vi "VI Interference Konfig.vi"() -> ()   [LabVIEW 2020, in "EPA 1065.lvlib" / "Interference verificaton 1065-366.lvlib"]
uses:
  Interference verificaton 1065-366.lvlib
  Visualisierungs Elemente/Zahlen-Ausgabefeld.ctl
  ResultTable.ctl
  TestKonfig.ctl
  Modus.ctl
  TestSetting.ctl
  Seiten/System Einstellungen V2/Analysatoren.ctl
  Visualisierungs Elemente/String - Ausgabefeld.ctl
  Aktion Test.ctl
  Aktion FGV Interference.ctl
  Sprachverwaltung/FGV Aktion Tabelle zerlegen.ctl
  Seiten/FT-IR/FGV FT-IR Gasliste Aktionen.ctl
  Aktion Index uebersetzten.ctl
  Allgemeine VIs/Aktion Test Status.ctl
  Allgemeine VIs/Aktion Wertaenderung Gasliste.ctl
  Messdaten/Aktionen FGV Messdaten.ctl
  Funktionstasten/Zustaende.ctl
  Funktionstasten/Funktionstasten-Aktion.ctl
  <vilib>/Utility/miscctls.llb/LVRowAndColumnTypeDef.ctl
  Seiten/FT-IR/FGV FT-IR Parameter.vi
  Messdaten/Messdaten.lvlib
  Seiten/Grafik/Grafik.lvlib
  Allgemein/allgemeine Sub-VIs.lvlib
  Seiten/FT-IR/FT-IR.lvlib
  Sprachverwaltung/Sprachverwaltung.lvlib
  Funktionstasten/Funktionstasten.lvlib
  Linearisierung V2/Protokoll/Protokoll.lvlib
  Seiten/FT-IR/Span/Spanfaktor.lvlib
  EPA 1065.lvlib
  Seiten/System Einstellungen V2/System Einstellungen V2.lvlib
panel:
  in  "Systemeinstellung":bool caption="Gasliste geändert"
  out "[%]":sgl=120.0 caption="Querempfindlichkeit:" min=0 format="%#.6g"
  in  "Gasliste vergleichen":bool
  in  "Registerkarte":T1(tab)
  in  "TestSetting":T2={"Bearbeiter:"="", "Pfad:"=path "D:/IAG_Data/Log", "Textname:"="", "Analysator"=""}
  in  "TestKonfig":T4={"CH4:"=0, "Ethane:"=0, "NMHC:"=0, "NMNEHC:"=0, "Komp 1 aktiv:"=FALSE, "Komp 2 aktiv:"=FALSE, "Komp 3 aktiv:"=FALSE, "Komp 4 aktiv:"=FALSE, "Modus"=0, "CG Aufschaltzeit:"=120.0, "Interferent 1: CO2"=0, "Interferent 2: H2O"=0, "Interferent 3: CH4"=0, "Interferent 4: C2H6 / C3H8"=0, "Gasflaschen Nr.:"="", "Gasflaschen Nr.: 3"="", "Gasflaschen Nr.: 4"="", "Inter 1 aktiv"=FALSE, "Inter 2 aktiv"=FALSE, "Inter 3 aktiv"=FALSE, "Inter 4 aktiv"=FALSE, "Accuracy"="", "Accuracy 3"="", "Accuracy 4"="", "Konzentration 1:"=120.0, "Konzentration 2:"=120.0, "Konzentration 3:"=120.0, "Konzentration 4:"=120.0, "Flow weighted mean 1:"=0.0, "Flow weighted mean 2:"=0.0, "Flow weighted mean 3:"=0.0, "Flow weighted mean 4:"=0.0} {"Flow weighted mean 4:" min=0.0; "NMNEHC:" items=["NMNEHCD (3000)"]; "Flow weighted mean 3:" min=0.0; "Flow weighted mean 2:" min=0.0; "Flow weighted mean 1:" min=0.0; "NMHC:" items=["NMHCD (10000)"]; "Ethane:" items=["Ethane (1000) LP 191C"]; "CH4:" items=["CH4 (250) LP 191C (1of2)", "CH4 (5000) LP 191C (2of2)", "CH4 autorange (5000)"]; "Konzentration 4:" min=0.0; "Interferent 4: C2H6 / C3H8" items=["Ethane (1000) LP 191C", "Propane (200) LP 191C"]; "Konzentration 3:" min=0.0; "Interferent 3: CH4" items=["CH4 (250) LP 191C (1of2)", "CH4 (5000) LP 191C (2of2)", "CH4 autorange (5000)"]; "Konzentration 2:" min=0.0; "Interferent 2: H2O" items=["H2O% (30) LP 191C", "H2Oppm (300000)"]; "Konzentration 1:" min=0.0; "Interferent 1: CO2" items=["CO2 low% (4) LP 191C (2of2)", "CO2% (20) LP 191C (1of2)", "CO2% autorange (20)"]; "Modus" items=["Messen", "CG zu Entnahmestelle"]; "CG Aufschaltzeit:" min=60.0}
  in  "Speichern":bool
  out "Komponente 4S:":T6 caption="NMNEHC:"
  out "Komponente 4:":T7 caption="ppm" format="%#.2f"
  out "Komponente 3S:":T6 caption="NMHC:"
  out "Komponente 3:":T7 caption="ppm" format="%#.2f"
  out "Komponente 2S:":T6 caption="Ethane:"
  out "Komponente 2:":T7 caption="ppm" format="%#.2f"
  in  "Graph löschen":bool caption="Test Start"
  out "Interferent 4:":T6 caption="Interferent 3:"
  out "Interferent 4:":T7 caption="ppm" format="%#.2f"
  out "Interferent 3:":T6
  out "Interferent 3: 2":T7 caption="ppm" format="%#.2f"
  out "Interferent 2:":T6
  out "Interferent 2: 2":T7 caption="%" format="%#.2f"
  out "Interferent 1:":T6
  out "Interferent 1: 2":T7 caption="%" format="%#.2f"
  in  "Abbrechen":bool caption="Test Start"
  out "Testdauer":T7
  out "Stabilisierungszeit":T7
  out "Graph":waveform(dbl)[](graph)
  out "Status":string
  in  "Test Start":bool
  out "Komponente 1S:":T6 caption="CH4:"
  out "Komponente 1:":T7 caption="ppm" format="%#.2f"
  in  "Save to file":bool caption="PDF erstellen"
  out "Grenze in ppm:":sgl=2.0 min=0 format="%#.6g"
  out "[%]":sgl=2.0 caption="Grenze:" min=0 format="%#.6g"
  out "Konzentration Komponente":sgl=120.0 caption="Konzentration:" min=0
  out "Komponente:":T6 caption="ppm"
  out "max. Flow Weighted Mean:":T6 caption="ppm"
  out "Konzentration FlowWeightedMean":sgl=120.0 caption="Konzentration:" min=0 format="%#.2f"
  out "LIN Ausgabetabelle":T8
  in  "Daten löschen":bool caption="Test Start"
  in  "Print to PDF":bool caption="PDF erstellen"
  out "Tabelle 3":string[][](table)
  # "HC Querempfindlichkeitsnachweis 1065.366"
  # "Interference Test"
  # "Interference Verification"
  # "Einstellungen"
  # "Allgemeine Einstellungen"
  # "Protocol Settings"
  # "Test Einstellungen"
  # "Durchflussgewichteter Mittelwert:"
  # "Interferenten"
  # "sec."
  # "Test"
  # "Ergebnis"
  # "Analyse"
  # "Interferenz für Komponente:"
  # "Durchflussgewichteter Mittelwert:"
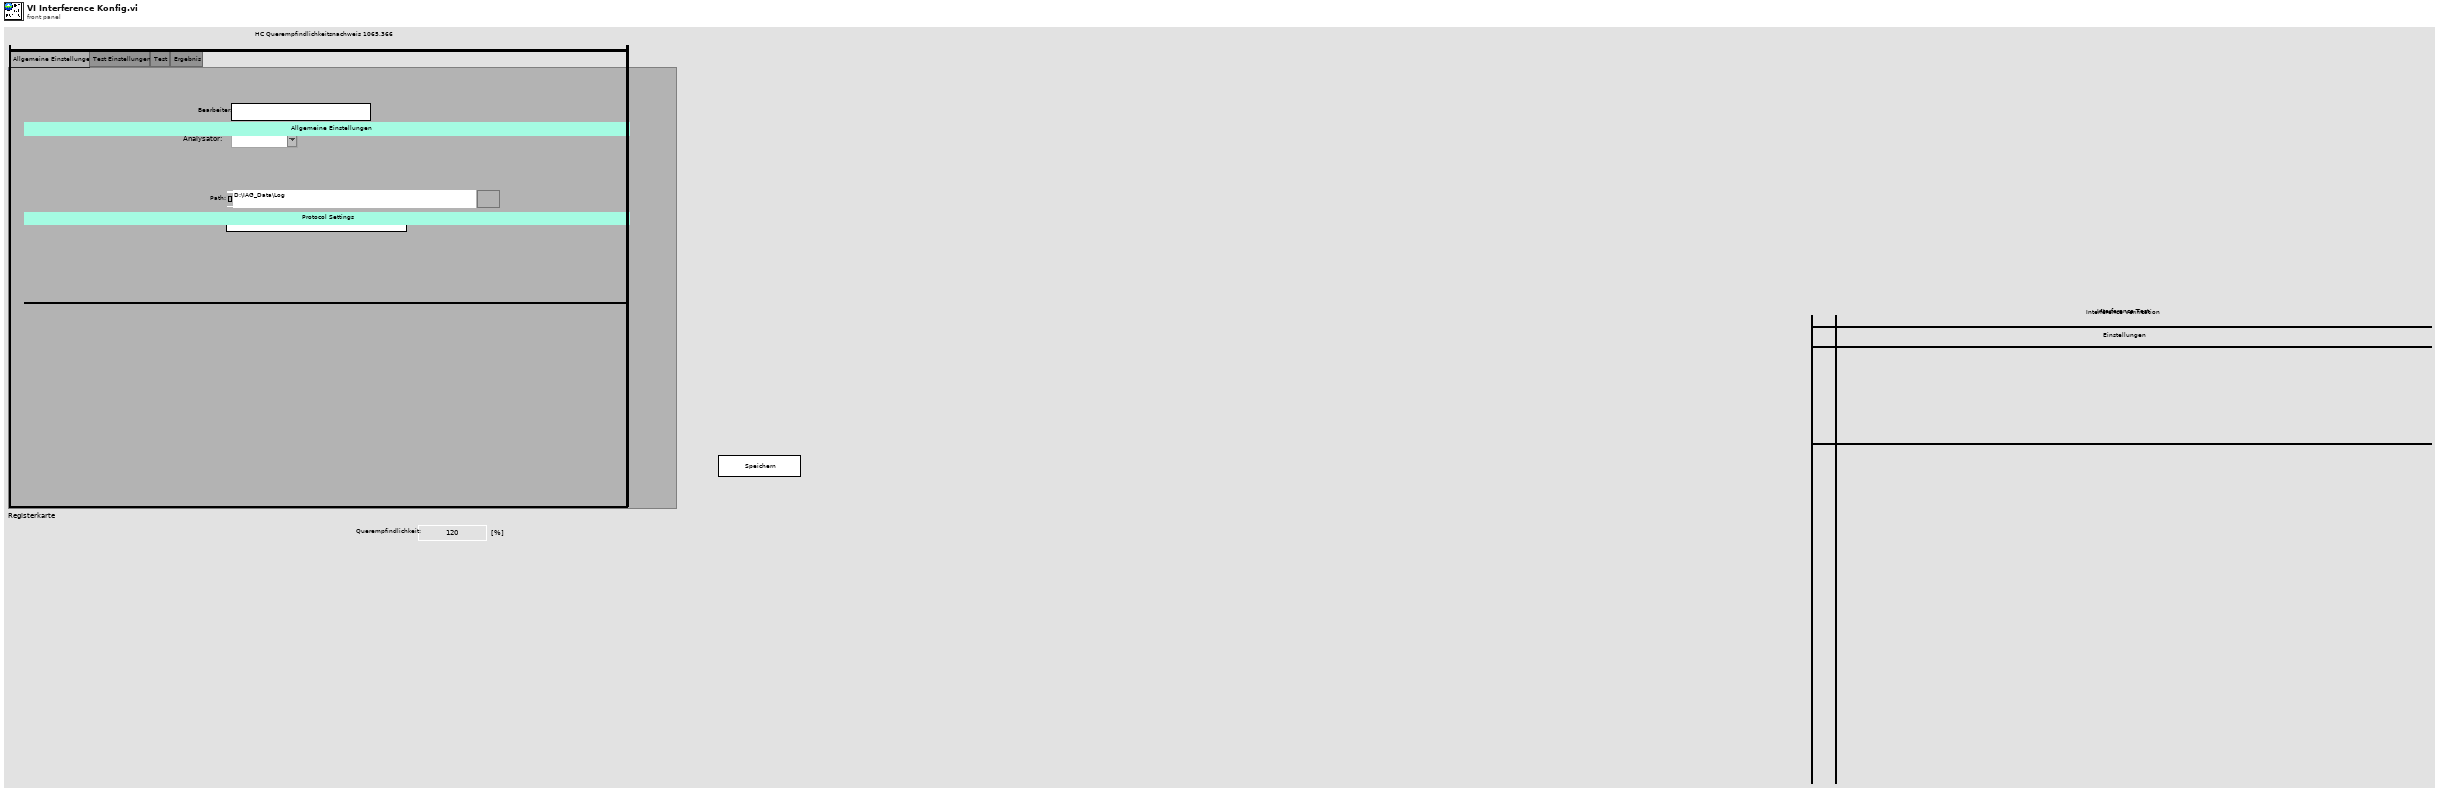
[diagram p1: front panel]
types:
  T1 = enum32{"General Settings", "Test Settings", "Test", "Result"}
  T2 = typedef "EPA 1065.lvlib/Interference verificaton 1065-366.lvlib/TestSetting.ctl" = cluster{"Bearbeiter:":string, "Pfad:":path, "Textname:":string, "Analysator":T3}
  T3 = typedef "System Einstellungen V2.lvlib/Analysatoren.ctl" = string
  T4 = typedef "EPA 1065.lvlib/Interference verificaton 1065-366.lvlib/TestKonfig.ctl" = cluster{"CH4:":u16, "Ethane:":u16, "NMHC:":u16, "NMNEHC:":u16, "Komp 1 aktiv:":bool, "Komp 2 aktiv:":bool, "Komp 3 aktiv:":bool, "Komp 4 aktiv:":bool, "Modus":T5, "CG Aufschaltzeit:":dbl, "Interferent 1: CO2":u16, "Interferent 2: H2O":u16, "Interferent 3: CH4":u16, "Interferent 4: C2H6 / C3H8":u16, "Gasflaschen Nr.:":string, "Gasflaschen Nr.: 3":string, "Gasflaschen Nr.: 4":string, "Inter 1 aktiv":bool, "Inter 2 aktiv":bool, "Inter 3 aktiv":bool, "Inter 4 aktiv":bool, "Accuracy":string, "Accuracy 3":string, "Accuracy 4":string, "Konzentration 1:":dbl, "Konzentration 2:":dbl, "Konzentration 3:":dbl, "Konzentration 4:":dbl, "Flow weighted mean 1:":dbl, "Flow weighted mean 2:":dbl, "Flow weighted mean 3:":dbl, "Flow weighted mean 4:":dbl}
  T5 = typedef "EPA 1065.lvlib/Interference verificaton 1065-366.lvlib/Modus.ctl" = u16
  T6 = typedef "String - Ausgabefeld.ctl" = string
  T7 = typedef "Zahlen-Ausgabefeld.ctl" = sgl
  T8 = typedef "EPA 1065.lvlib/Interference verificaton 1065-366.lvlib/ResultTable.ctl" = string[][]
  T9 = typedef "EPA 1065.lvlib/Interference verificaton 1065-366.lvlib/Aktion Test.ctl" = enum16{"Lesen", "ini", "ini - Konz", "Konzentration erreicht", "ini-warten", "ini-Warten-Stabil", "Warten-Stabil", "ini-warten-aufzeichnen", "Warten-Aufzeichnen", "aufzeichnen", "ini-wet", "ini - konz - wet", "Konzentration erreicht - wet", "ini - warten - wet", "warten - wet", "warten - aufzeichnen - wet", "Auswerten", "aufzeichnen - wet"}
  T10 = typedef "Sprachverwaltung.lvlib/FGV Aktion Tabelle zerlegen.ctl" = enum16{"laden", "vereinzeln", "speichern"}
  T11 = typedef "EPA 1065.lvlib/Interference verificaton 1065-366.lvlib/Aktion FGV Interference.ctl" = enum16{"Lesen", "TestKonfig", "TestSetting", "Einheiten", "Ergebnis", "Laden", "Tabelle", "Speichern", "löschen"}
  T12 = enum16{"Deutsch", "Englisch", "Französisch", "Italienisch"}
  T13 = enum8{"Enabled", "Disabled", "Disabled and Grayed Out"}
  T14 = typedef "EPA 1065.lvlib/Interference verificaton 1065-366.lvlib/Aktion Index uebersetzten.ctl" = enum16{"lesen", "schreiben", "auswerten"}
  T15 = typedef "FT-IR.lvlib/FGV FT-IR Gasliste Aktionen.ctl" = enum16{"lesen", "Gasliste FT-IR", "Gasliste ausgelesen", "laden", "speichern", "löschen"}
  T16 = typedef "EPA 1065.lvlib/Interference verificaton 1065-366.lvlib/Komponenten.ctl" = cluster{"Komponente":T6, "Komponente Index":i32, "Komponente 2":T6, "Komponente Index 2":i32, "Komponente 3":T6, "Komponente Index 3":i32, "Komponente 4":T6, "Komponente Index 4":i32, "Interferent 1":T6, "Interferent Index":i32, "Interferent 2":T6, "Interferent 2 Index":i32, "Interferent 3":T6, "Interferent 3 Index":i32, "Interferent 4":T6, "Interferent 4 Index":i32}
  T17 = typedef "EPA 1065.lvlib/Aktion Wertaenderung Gasliste.ctl" = enum16{"Init", "lesen", "Gasliste geändert", "ARN inaktiv", "LEAK inaktiv", "Interference 366 inaktiv", "T90 inaktiv", "Interference 375 inaktiv", "Chiller inaktiv", "FID O2 inaktiv", "FID Opti inaktiv", "Drift inaktiv", "Pre Test inaktiv", "LinV2 inaktiv", "HovaCAL Interference inaktiv"}
  T18 = typedef "EPA 1065.lvlib/Aktion Test Status.ctl" = enum16{"init", "lesen", "prüfen", "Interference 366", "Interference 375", "Chiller läuft", "Drift läuft", "Pre Test läuft", "FID Optimization läuft", "FID Interference läuft", "HovaCAL Interference", "LinV2"}
  T19 = typedef "Messdaten.lvlib/Aktionen FGV Messdaten.ctl" = enum16{"lesen", "schreiben", "löschen", "Mittelwerte", "Komponente"}
  T20 = typedef "Funktionstasten.lvlib/Funktionstasten-Aktion.ctl" = enum16{"Initialisieren", "Zustand setzen", "Taste gedrückt", "Fehler speichern", "Lesen", "Manuell", "Remote", "Bitparallel", "Samplepoint", "Zeit Prüfen", "reset Umschalten"}
  T21 = typedef "Funktionstasten.lvlib/Zustaende.ctl" = enum16{"Standby", "Pause", "Eco", "Messen", "Kalibrieren", "Spülen Filter", "Spülen Leitung", "Umgebungsluft", "0-Gas", "Cal-Gas", "CG zu PNS", "-------------", "Init 1", "Init 2", "Init 3", "Init 4", "Messen vorbereiten", "Messen durchführen", "Exit"}
  T22 = enum16{"open", "replace", "create", "open or create", "replace or create", "replace or create with confirmation"}
  T23 = typedef "LVRowAndColumnTypeDef.ctl" = cluster{"Row":i32, "Column":i32}
  T24 = typedef "EPA 1065.lvlib/Aktive Tests Cluster.ctl" = cluster{"ANR läuft":bool, "T90 läuft":bool, "Leak läuft":bool, "Interference 366 läuft":bool, "Interference 375 läuft":bool, "Chiller läuft":bool, "FID Interference läuft":bool, "FID optimization läuft":bool, "Drift läuft":bool, "Pre-test läuft":bool, "HovaCAL Interference läuft":bool, "LinV2 läuft":bool}
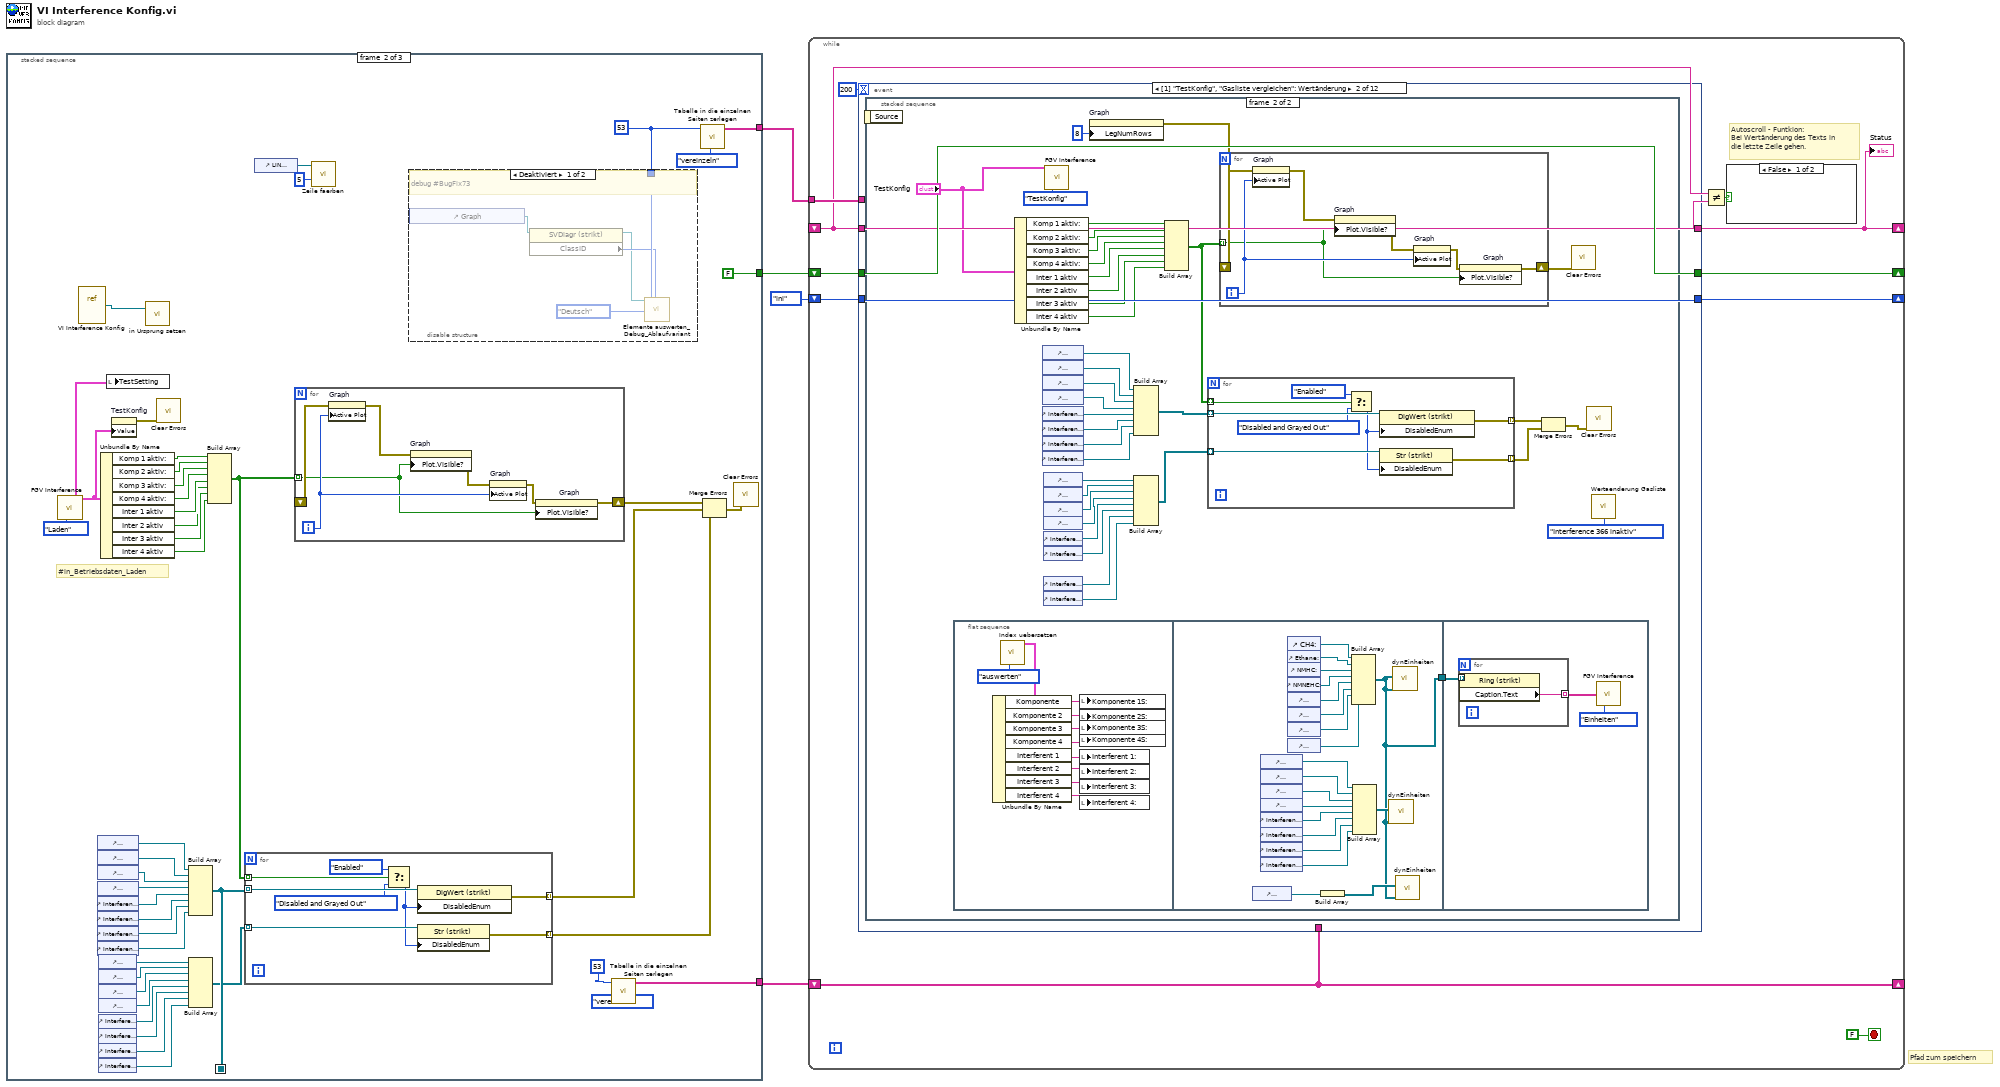
[diagram p0: block diagram]
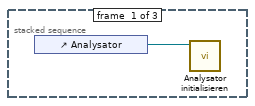
[diagram p2: hidden frame]
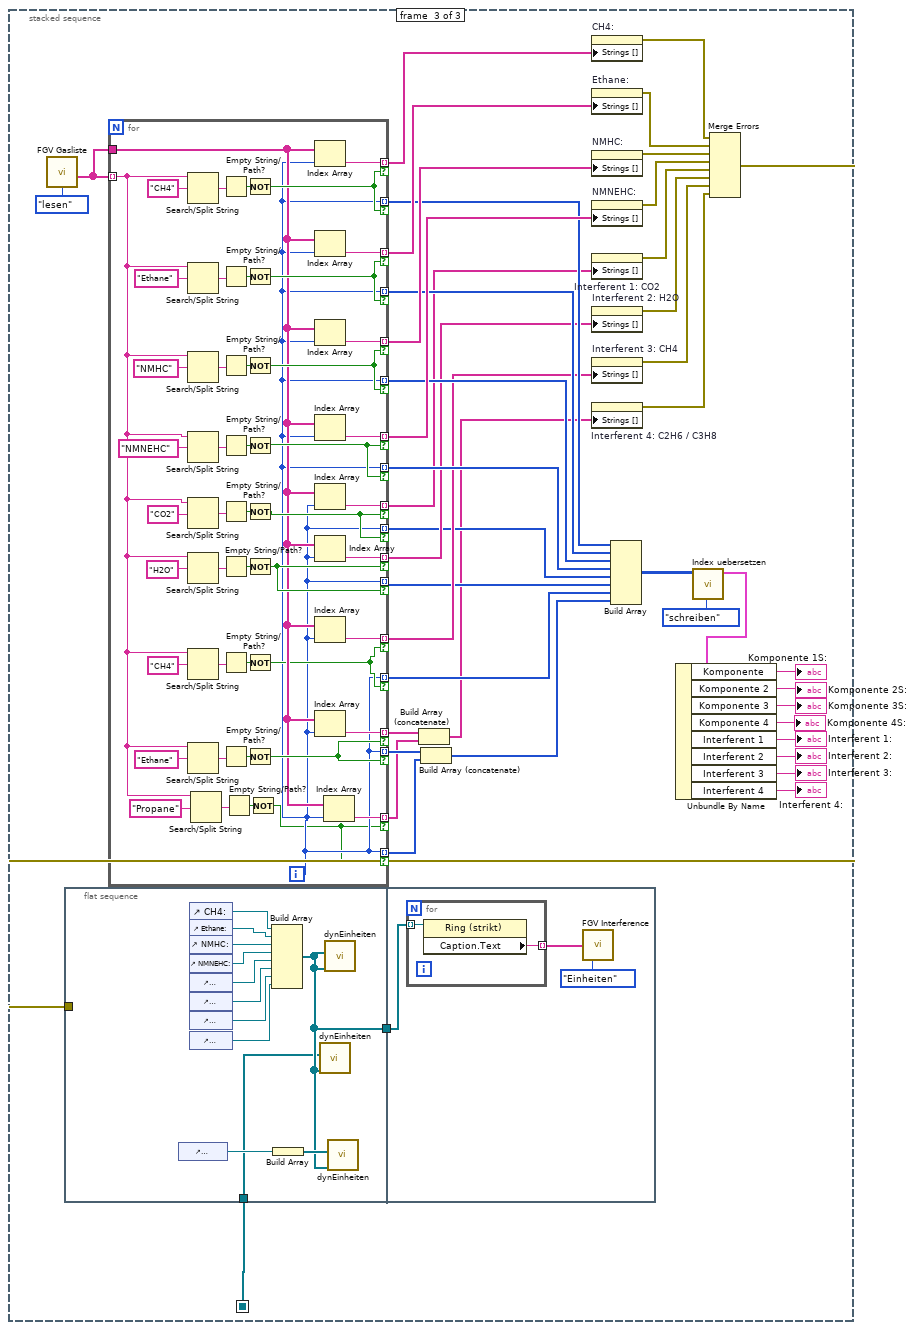
[diagram p4: hidden frame]
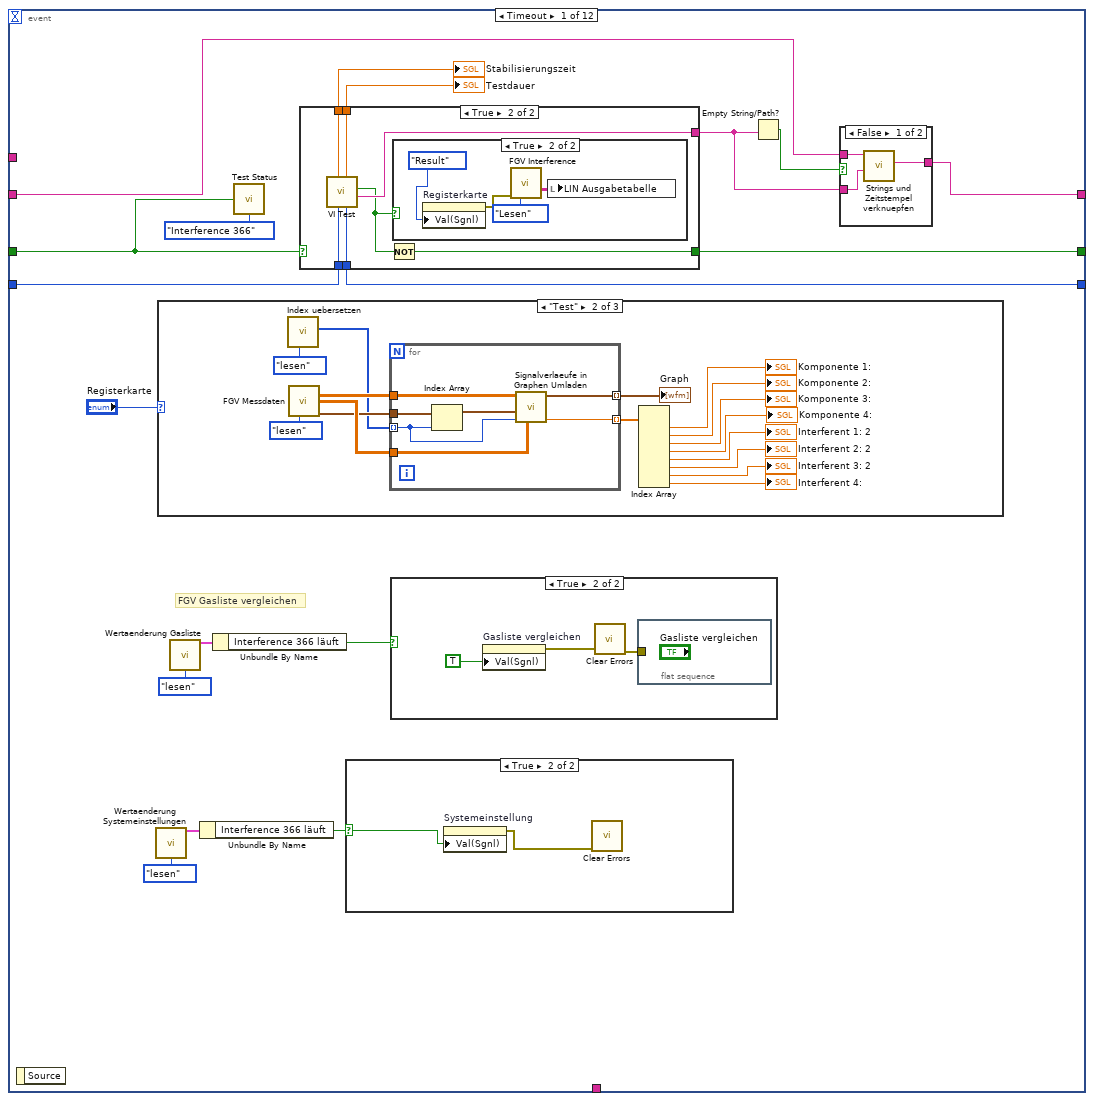
[diagram p5: hidden frame]
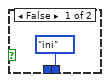
[diagram p10: hidden frame]
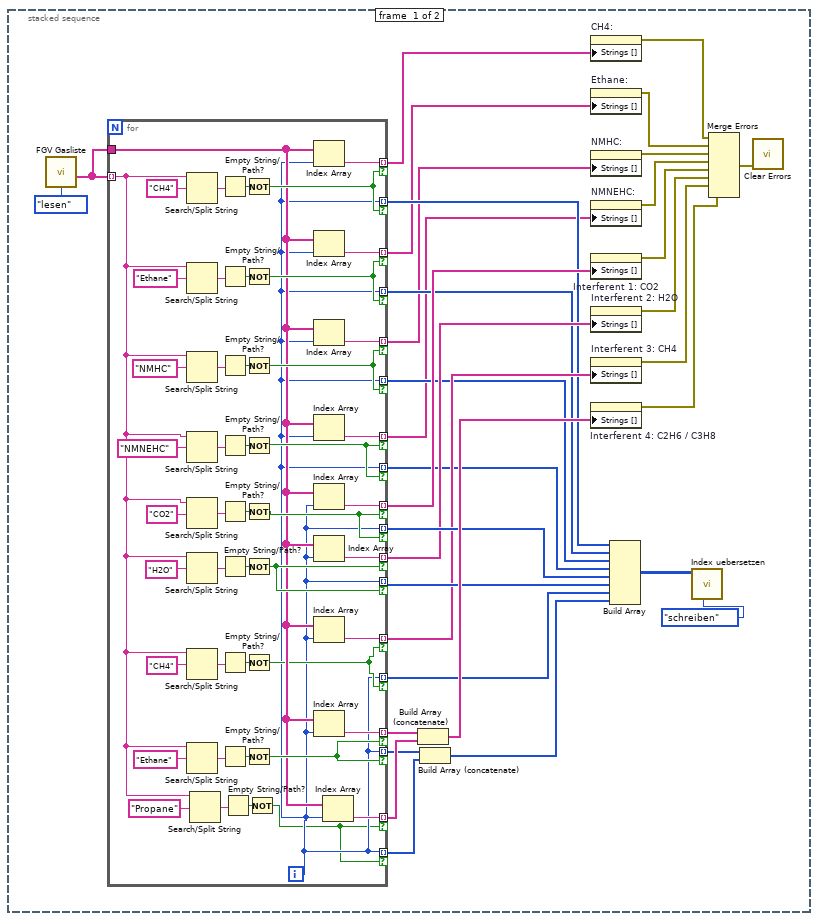
[diagram p13: hidden frame]
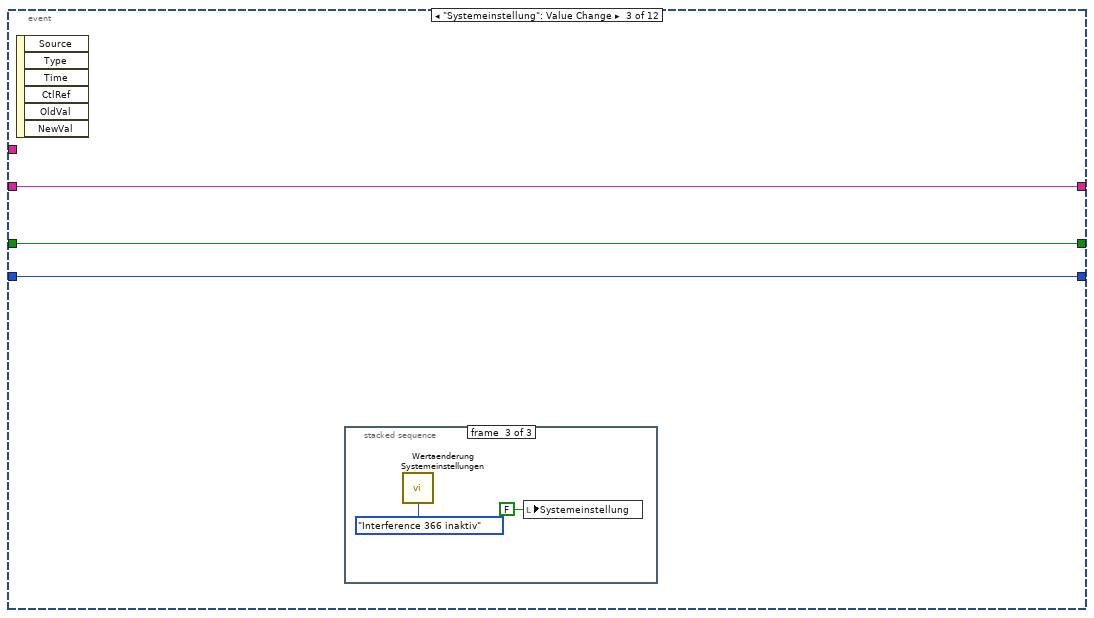
[diagram p14: hidden frame]
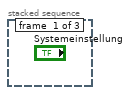
[diagram p15: hidden frame]
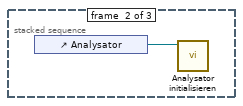
[diagram p16: hidden frame]
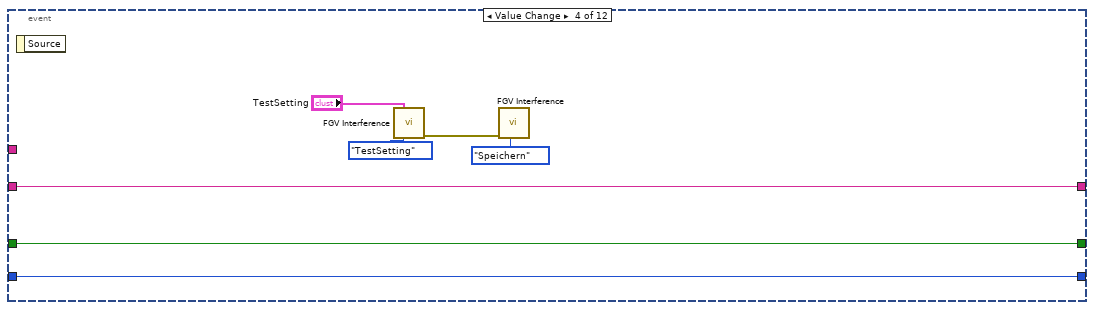
[diagram p17: hidden frame]
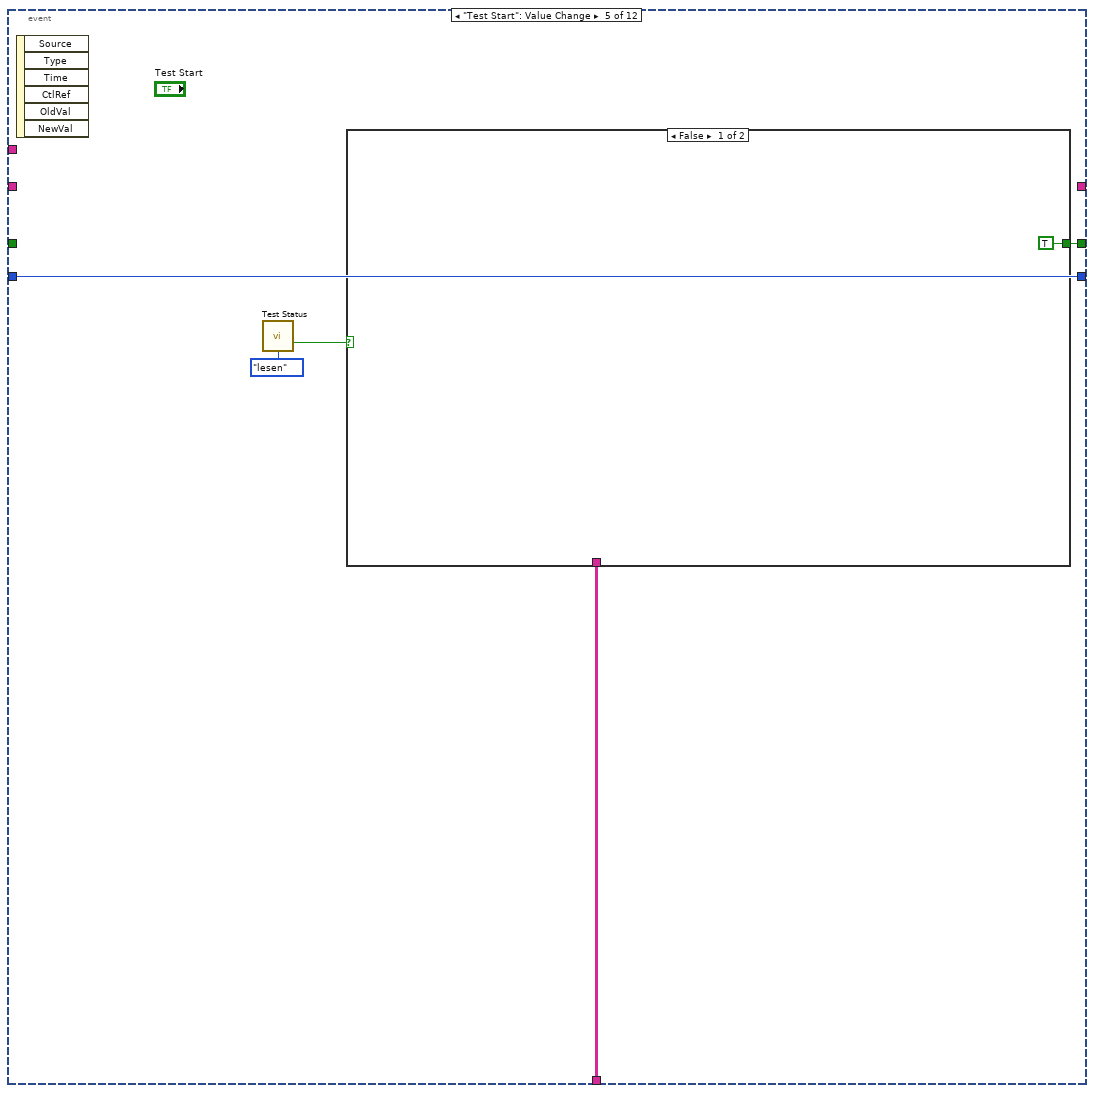
[diagram p18: hidden frame]
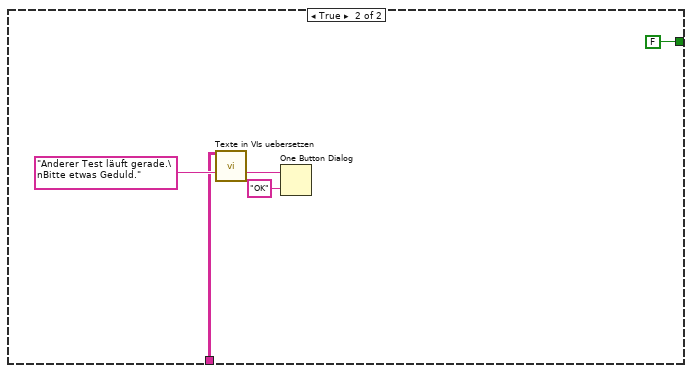
[diagram p19: hidden frame]
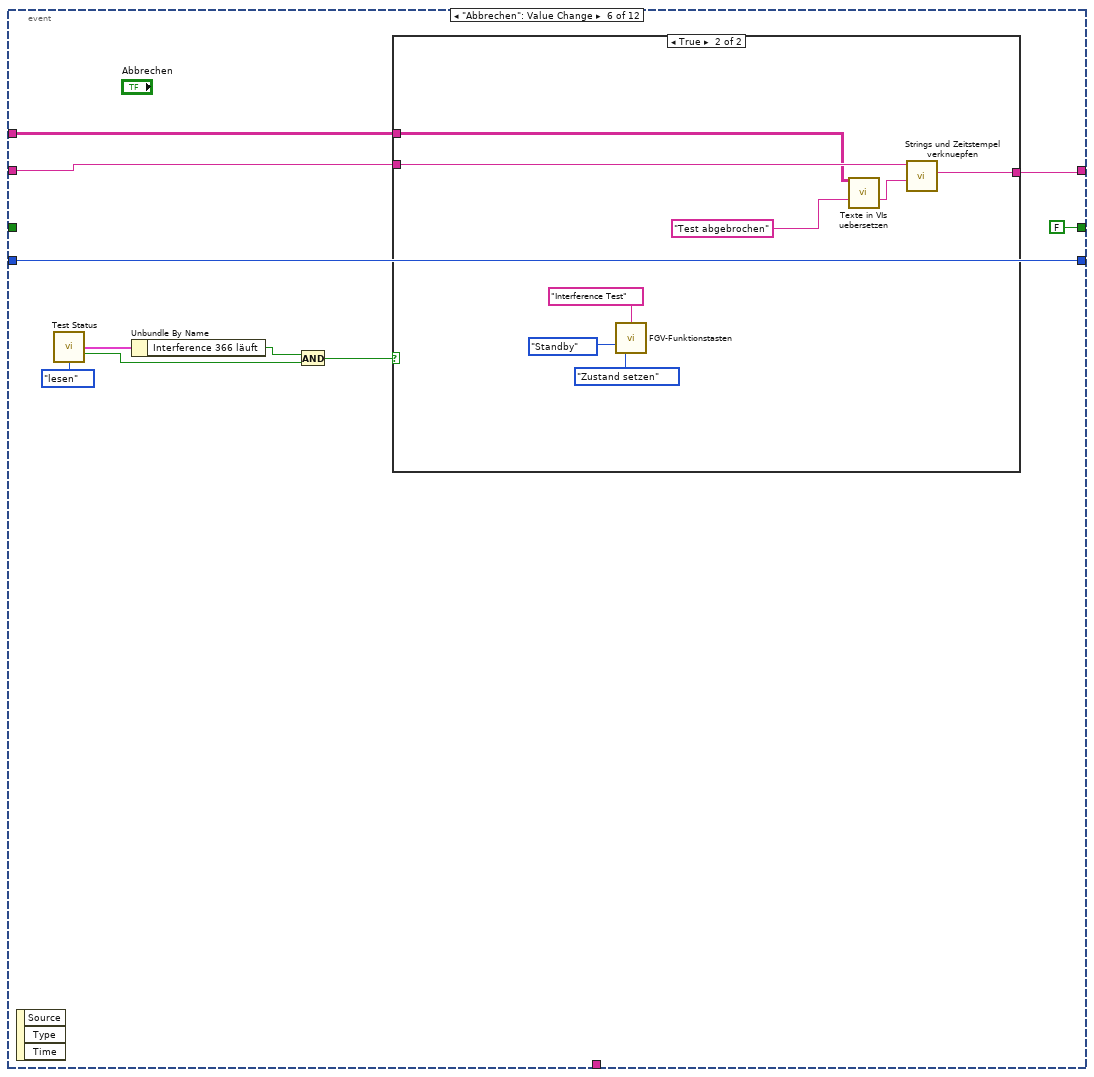
[diagram p20: hidden frame]
diagram:
  # "Pfad zum speichern"
  n1 = stacked-sequence {
    seq-local: [_ w15 _] -> [_ _ w93]
    tunnel: [_ w50 _] -> w4
    tunnel: [_ FALSE _] -> w3
    tunnel: [_ w31 _] -> w1
    frame #0 {
      n2 = control-ref of="Analysator"() -> (w5:refnum<vi>)
      n3 = call "Analysator initialisieren.vi"("Referenz Analysator"=w5) -> ()  [unwired: 9 in, 2 out]
    }
    frame #1 {
      w7 = 53 ("Index (Seite)")
      # "#in_Betriebsdaten_Laden"
      n4 = call "FGV Interference.vi"("Aktion FGV Interference"=Aktion_FGV_Interference."Laden") -> ("TestSetting"=w43:T2, "TestKonfig"=w47:T4)  [unwired: 9 in, 4 out]
      n5 = vi-ref "VI Interference Konfig.vi"() -> (w30:refnum<vi>)
      n6 = control-ref of="Komponente 1:"() -> (w20:refnum<vi>)
      n7 = control-ref of="Komponente 2:"() -> (w21:refnum<vi>)
      n8 = control-ref of="Komponente 3:"() -> (w22:refnum<vi>)
      n9 = control-ref of="Komponente 4:"() -> (w9:refnum<vi>)
      n10 = control-ref of="Interferent 1: 2"() -> (w18:refnum<vi>)
      n11 = control-ref of="Interferent 2: 2"() -> (w17:refnum<vi>)
      n12 = control-ref of="Interferent 3: 2"() -> (w16:refnum<vi>)
      n13 = control-ref of="Interferent 3: 3"() -> (w19:refnum<vi>)
      n14 = control-ref of="Komponente 1S:"() -> (w23:refnum<vi>)
      n15 = control-ref of="Komponente 2S:"() -> (w24:refnum<vi>)
      n16 = control-ref of="Komponente 3S:"() -> (w25:refnum<vi>)
      n17 = control-ref of="Komponente 4S:"() -> (w8:refnum<vi>)
      n18 = control-ref of="Interferent 1:"() -> (w26:refnum<vi>)
      n19 = control-ref of="Interferent 2:"() -> (w27:refnum<vi>)
      n20 = control-ref of="Interferent 3:"() -> (w28:refnum<vi>)
      n21 = control-ref of="Interferent 4:"() -> (w29:refnum<vi>)
      n22 = Unbundle By Name(w47) -> ("Komp 1 aktiv:"=w42:bool, "Komp 2 aktiv:"=w41:bool, "Komp 3 aktiv:"=w40:bool, "Komp 4 aktiv:"=w10:bool, "Inter 1 aktiv"=w39:bool, "Inter 2 aktiv"=w34:bool, "Inter 3 aktiv"=w38:bool, "Inter 4 aktiv"=w37:bool)
      n23 = local write "TestSetting"(w43) -> ()
      n24 = property on="TestKonfig" class="Cluster (strikt)"("Value"=w47) -> (error out=w46:errorcluster)  [unwired: 2 in, 1 out]
      n25 = call "in Ursprung setzen.vi"("VI Referenz"=w30) -> ()  [unwired: 10 in, 1 out]
      n26 = call <vilib>:"Clear Errors.vi"("error in (no error)"=w46) -> ()  [unwired: 5 in, 2 out]
      n27 = Build Array(w20, w21, w22, w9, w18, w17, w16, w19) -> (w15:refnum<vi>[])
      n28 = Build Array(w23, w24, w25, w8, w26, w27, w28, w29) -> (w14:refnum<vi>[])
      n29 = Build Array(w42, w41, w40, w10, w39, w34, w38, w37) -> (w13:bool[])
      n30 = for {
        tunnel: w13 -> [w56] mode=indexing
        tunnel: w15 -> [w63] mode=indexing
        tunnel: w14 -> [w62] mode=indexing
        tunnel: [w61] -> w12 mode=indexing
        tunnel: [w60] -> w11 mode=indexing
        n31 = Select(t=T13."Enabled" ("Deaktiviert"), s=w56, f=T13."Disabled and Grayed Out" ("Deaktiviert")) -> (s? t:f=w57:T13)
        n32 = property class="DigWert (strikt)"(reference=w63, "DisabledEnum"=w57) -> (error out=w61:errorcluster)  [unwired: 1 in, 1 out]
        n33 = property class="Str (strikt)"(reference=w62, "DisabledEnum"=w57) -> (error out=w60:errorcluster)  [unwired: 1 in, 1 out]
      }
      n34 = control-ref of="LIN Ausgabetabelle"() -> (w44:refnum<vi>)
      n35 = for {
        shift-right: [w67] -> w36
        shift-left: _ -> [w66]
        tunnel: w13 -> [w64] mode=indexing
        i -> [w65]
        n36 = property on="Graph" class="SVDiagr (strikt)"(error in=w66, "Active Plot"=w65) -> (error out=w68:errorcluster)  [unwired: 1 in, 1 out]
        n37 = property on="Graph" class="SVDiagr (strikt)"(error in=w68, "Plot.Visible?"=w64) -> (error out=w69:errorcluster)  [unwired: 1 in, 1 out]
        n38 = property on="Graph" class="SVDiagr (strikt)"(error in=w69, "Active Plot"=w65) -> (error out=w70:errorcluster)  [unwired: 1 in, 1 out]
        n39 = property on="Graph" class="SVDiagr (strikt)"(error in=w70, "Plot.Visible?"=w64) -> (error out=w67:errorcluster)  [unwired: 1 in, 1 out]
      }
      n40 = call "Zeile faerben.vi"("Anzahl"=5, "Table (Eingang)"=w44) -> ()  [unwired: 9 in, 1 out]
      n41 = disable-structure shown="Deaktiviert" {
        disable-tunnel: w7 -> [w55 _]
        frame Disabled {
          # "debug #BugFix73"
          n42 = control-ref of="Graph"() -> (w52:refnum<vi>)
          n43 = property class="SVDiagr (strikt)"(reference=w52) -> (reference out=w51:refnum<vi>, "ClassID"=w54:u32)  [unwired: 1 in, 1 out]
          n44 = call "Elemente auswerten_Debug_Ablaufvariant.vi"("GObject (Eingang)"=w51, "Sprachauswahl"=T12."Deutsch", "Index"=w55, "ClassID"=w54) -> ()  [unwired: 13 in, 3 out]
        }
        frame Enabled {
        }
      }
      n45 = call "Tabelle in die einzelnen Seiten zerlegen.vi"("Aktion"=FGV_Aktion_Tabelle_zerlegen."vereinzeln", "Index (Seite)"=53) -> ("Sprachliste"=w31:string[][])  [unwired: 7 in, 2 out]
      n46 = call "Tabelle in die einzelnen Seiten zerlegen.vi"("Aktion"=FGV_Aktion_Tabelle_zerlegen."vereinzeln", "Index (Seite)"=w7) -> ("Sprachliste"=w50:string[][])  [unwired: 7 in, 2 out]
      n47 = Merge Errors(w36, w12, w11) -> (w35:errorcluster)
      n48 = call <vilib>:"Clear Errors.vi"("error in (no error)"=w35) -> ()  [unwired: 5 in, 2 out]
    }
    frame #2 {
      n49 = call "FGV Gasliste.vi"("Aktionen"=FGV_FT-IR_Gasliste_Aktionen."lesen") -> ("Aktuelle Gasliste gesamt"=w112:T6[])  [unwired: 8 in, 2 out]
      n50 = flat-sequence {
        tunnel: w111 -> [_]
        tunnel: [w119] -> w114
        tunnel: w93 -> [w116]
        tunnel: w114 -> [w129]
        frame #0 {
          n51 = control-ref of="Komponente:"() -> (w121:refnum<vi>)
          n52 = control-ref of="CH4:"() -> (w118:refnum<vi>)
          n53 = control-ref of="Ethane:"() -> (w117:refnum<vi>)
          n54 = control-ref of="NMHC:"() -> (w126:refnum<vi>)
          n55 = control-ref of="NMNEHC:"() -> (w125:refnum<vi>)
          n56 = control-ref of="Interferent 1: CO2"() -> (w124:refnum<vi>)
          n57 = control-ref of="Interferent 2: H2O"() -> (w123:refnum<vi>)
          n58 = control-ref of="Interferent 3: CH4"() -> (w120:refnum<vi>)
          n59 = control-ref of="Interferent 3: CH4"() -> (w115:refnum<vi>)
          n60 = Build Array(w118, w117, w126, w125, w124, w123, w120, w115) -> (w119:refnum<vi>[])
          n61 = Build Array(w121) -> (w122:refnum<vi>[])
          n62 = call "dynEinheiten.vi"("Komponenten Ref."=w119, "Sollwert Ref."=w116) -> ()  [unwired: 10 in]
          n63 = call "dynEinheiten.vi"("Komponenten Ref."=w119, "Sollwert Ref."=w119) -> ()  [unwired: 10 in]
          n64 = call "dynEinheiten.vi"("Komponenten Ref."=w119, "Sollwert Ref."=w122) -> ()  [unwired: 10 in]
        }
        frame #1 {
          n65 = for {
            tunnel: w129 -> [w131] mode=indexing
            tunnel: [w130] -> w127 mode=indexing
            n66 = property class="Ring (strikt)"(reference=w131) -> ("Caption.Text"=w130:string)  [unwired: 1 in, 2 out]
          }
          n67 = call "FGV Interference.vi"("Êinheiten"=w127, "Aktion FGV Interference"=Aktion_FGV_Interference."Einheiten") -> ()  [unwired: 8 in, 6 out]
        }
      }
      n68 = for {
        tunnel: w112 -> [w137] mode=indexing
        tunnel: w112 -> [w136]
        tunnel: [w176] -> w92 mode=indexing if=w175
        tunnel: [w133] -> w88 mode=indexing if=w175
        tunnel: [w173] -> w91 mode=indexing if=w174
        tunnel: [w133] -> w87 mode=indexing if=w174
        tunnel: [w166] -> w90 mode=indexing if=w165
        tunnel: [w133] -> w86 mode=indexing if=w165
        tunnel: [w163] -> w83 mode=indexing if=w164
        tunnel: [w133] -> w79 mode=indexing if=w164
        tunnel: [w156] -> w82 mode=indexing if=w134
        tunnel: [w133] -> w78 mode=indexing if=w134
        tunnel: [w155] -> w81 mode=indexing if=w142
        tunnel: [w149] -> w89 mode=indexing if=w148
        tunnel: [w133] -> w85 mode=indexing if=w148
        tunnel: [w144] -> w84 mode=indexing if=w143
        tunnel: [w133] -> w80 mode=indexing if=w143
        tunnel: [w133] -> w77 mode=indexing if=w142
        tunnel: [w135] -> w73 mode=indexing if=w132
        tunnel: [w133] -> w71 mode=indexing if=w132
        i -> [w133]
        n69 = Search/Split String(string=w137, search string/char (-)="CH4" ("Such-String/-Zeichen (-)")) -> (match + rest of string=w178:T6)  [unwired: 1 in, 2 out]
        n70 = Search/Split String(string=w137, search string/char (-)="Ethane" ("Such-String/-Zeichen (-)")) -> (match + rest of string=w171:T6)  [unwired: 1 in, 2 out]
        n71 = Search/Split String(string=w137, search string/char (-)="NMHC" ("Such-String/-Zeichen (-)")) -> (match + rest of string=w168:T6)  [unwired: 1 in, 2 out]
        n72 = Search/Split String(string=w137, search string/char (-)="NMNEHC" ("Such-String/-Zeichen (-)")) -> (match + rest of string=w151:T6)  [unwired: 1 in, 2 out]
        n73 = Search/Split String(string=w137, search string/char (-)="CO2" ("Such-String/-Zeichen (-)")) -> (match + rest of string=w146:T6)  [unwired: 1 in, 2 out]
        n74 = Search/Split String(string=w137, search string/char (-)="H2O" ("Such-String/-Zeichen (-)")) -> (match + rest of string=w161:T6)  [unwired: 1 in, 2 out]
        n75 = Search/Split String(string=w137, search string/char (-)="CH4" ("Such-String/-Zeichen (-)")) -> (match + rest of string=w158:T6)  [unwired: 1 in, 2 out]
        n76 = Search/Split String(string=w137, search string/char (-)="Ethane" ("Such-String/-Zeichen (-)")) -> (match + rest of string=w153:T6)  [unwired: 1 in, 2 out]
        n77 = Search/Split String(string=w137, search string/char (-)="Propane" ("Such-String/-Zeichen (-)")) -> (match + rest of string=w139:T6)  [unwired: 1 in, 2 out]
        n78 = Empty String/Path?(string/path=w178) -> (empty?=w179:bool)
        n79 = Empty String/Path?(string/path=w171) -> (empty?=w170:bool)
        n80 = Empty String/Path?(string/path=w168) -> (empty?=w169:bool)
        n81 = Empty String/Path?(string/path=w151) -> (empty?=w150:bool)
        n82 = Empty String/Path?(string/path=w146) -> (empty?=w147:bool)
        n83 = Empty String/Path?(string/path=w161) -> (empty?=w160:bool)
        n84 = Empty String/Path?(string/path=w158) -> (empty?=w159:bool)
        n85 = Empty String/Path?(string/path=w153) -> (empty?=w152:bool)
        n86 = Empty String/Path?(string/path=w139) -> (empty?=w138:bool)
        n87 = Not(x=w179) -> (.not. x?=w175:bool)
        n88 = Not(x=w170) -> (.not. x?=w174:bool)
        n89 = Not(x=w169) -> (.not. x?=w165:bool)
        n90 = Not(x=w150) -> (.not. x?=w148:bool)
        n91 = Not(x=w147) -> (.not. x?=w143:bool)
        n92 = Not(x=w160) -> (.not. x?=w164:bool)
        n93 = Not(x=w159) -> (.not. x?=w134:bool)
        n94 = Not(x=w152) -> (.not. x?=w142:bool)
        n95 = Not(x=w138) -> (.not. x?=w132:bool)
        n96 = Index Array(array=w136, index=w133) -> (element=w176:T6)
        n97 = Index Array(array=w136, index=w133) -> (element=w173:T6)
        n98 = Index Array(array=w136, index=w133) -> (element=w166:T6)
        n99 = Index Array(array=w136, index=w133) -> (element=w149:T6)
        n100 = Index Array(array=w136, index=w133) -> (element=w144:T6)
        n101 = Index Array(array=w136, index=w133) -> (element=w163:T6)
        n102 = Index Array(array=w136, index=w133) -> (element=w156:T6)
        n103 = Index Array(array=w136, index=w133) -> (element=w155:T6)
        n104 = Index Array(array=w136, index=w133) -> (element=w135:T6)
      }
      n105 = Build Array (concatenate)(w81, w73) -> (w74:T6[])
      n106 = Build Array (concatenate)(w77, w71) -> (w72:i32[])
      n107 = property on="CH4:" class="Ring (strikt)"("Strings []"=w92) -> (error out=w98:errorcluster)  [unwired: 2 in, 1 out]
      n108 = property on="Ethane:" class="Ring (strikt)"("Strings []"=w91) -> (error out=w97:errorcluster)  [unwired: 2 in, 1 out]
      n109 = property on="NMHC:" class="Ring (strikt)"("Strings []"=w90) -> (error out=w107:errorcluster)  [unwired: 2 in, 1 out]
      n110 = property on="NMNEHC:" class="Ring (strikt)"("Strings []"=w89) -> (error out=w108:errorcluster)  [unwired: 2 in, 1 out]
      n111 = property on="Interferent 1: CO2" class="Ring (strikt)"("Strings []"=w84) -> (error out=w109:errorcluster)  [unwired: 2 in, 1 out]
      n112 = property on="Interferent 2: H2O" class="Ring (strikt)"("Strings []"=w83) -> (error out=w110:errorcluster)  [unwired: 2 in, 1 out]
      n113 = property on="Interferent 3: CH4" class="Ring (strikt)"("Strings []"=w82) -> (error out=w100:errorcluster)  [unwired: 2 in, 1 out]
      n114 = property on="Interferent 4: C2H6 / C3H8" class="Ring (strikt)"("Strings []"=w74) -> (error out=w76:errorcluster)  [unwired: 2 in, 1 out]
      n115 = Build Array(w88, w87, w86, w85, w80, w79, w78, w72) -> (w113:i32[][])
      n116 = call "Index uebersetzen.vi"("Aktion"=Aktion_Index_uebersetzten."schreiben", "Array"=w113) -> ("Komponenten"=w104:T16)  [unwired: 8 in, 1 out]
      n117 = Unbundle By Name(w104) -> ("Komponente"=→"Komponente 1S:":T6, "Komponente 2"=→"Komponente 2S:":T6, "Komponente 3"=→"Komponente 3S:":T6, "Komponente 4"=→"Komponente 4S:":T6, "Interferent 1"=→"Interferent 1:":T6, "Interferent 2"=→"Interferent 2:":T6, "Interferent 3"=→"Interferent 3:":T6, "Interferent 4"=→"Interferent 4:":T6)
      n118 = Merge Errors(w98, w97, w107, w108, w109, w110, w100, w76) -> (w111:errorcluster)
    }
  }
  n119 = while {
    shift-right: [w187] -> _
    shift-left: w3 -> [w188]
    shift-right: [w183] -> _
    shift-left: _ -> [w185]
    tunnel: w4 -> [w186]
    shift-right: [w182] -> _
    shift-left: Aktion_Test."ini" ("Aktion") -> [w181]
    shift-right: [w180] -> _
    shift-left: w1 -> [w180]
    stop <- FALSE stop-if-true
    # "Autoscroll - Funtkion:\nBei Wertänderung des Texts in \ndie letzte Zeile gehen."
    n120 = event shown="[1] \"TestKonfig\", \"Gasliste vergleichen\": Wertänderung" {
      selector: _ -> [_ _ _ _ _ _ _ _ _ _ _ _]
      dyn-events: _ -> [_ _ _ _ _ _ _ _ _ _ _ _]
      timeout: 200 -> [_ _ _ _ _ _ _ _ _ _ _ _]
      tunnel: [w206 w253 w426 w432 _ w457 _ w492 w506 w528 w532 w538] -> w183
      tunnel: w185 -> [w205 w253 w426 w432 _ w456 _ w492 w506 w528 w532 w538]
      tunnel: w188 -> [w197 w255 w425 w433 _ _ w468 w491 w505 w530 w534 w553]
      tunnel: [w202 w255 w425 w433 w441 FALSE w468 w491 w505 w530 w534 w553] -> w187
      tunnel: w186 -> [_ _ _ _ _ w453 _ _ _ _ _ w540]
      tunnel: [w204 w254 w424 w434 w440 w455 w467 w490 w504 w529 w533 w554] -> w182
      tunnel: w181 -> [w203 w254 w424 w434 w440 w455 w467 w490 w504 w529 w533 w554]
      tunnel: w180 -> [_ _ _ _ w438 _ _ _ _ _ _ _]
      event Timeout {
        # "FGV Gasliste vergleichen"
        n121 = event-data() -> ()  [unwired: 1 in, 1 out]
        n122 = call "Wertaenderung Systemeinstellungen.vi"("Aktion"=Aktion_Wertaenderung_Gasliste."lesen") -> ("Tests"=w191:T24)  [unwired: 13 in, 1 out]
        n123 = case shown="\"Test\"" "Registerkarte" {
          frame "General Settings", Default {
          }
          frame "Test" {
            n124 = call "Index uebersetzen.vi"("Aktion"=Aktion_Index_uebersetzten."lesen") -> ("Komponenten"=w224:i32[])  [unwired: 9 in, 1 out]
            n125 = call "FGV Messdaten.vi"("Aktionen"=Aktionen_FGV_Messdaten."lesen") -> ("Messdaten"=w225:sgl[][], "Mittelwertdaten"=w227:sgl[][], "Zeitstempeln"=w226:timestamp[])  [unwired: 6 in, 6 out]
            n126 = for {
              tunnel: w227 -> [w236]
              tunnel: w226 -> [w235]
              tunnel: w225 -> [w233]
              tunnel: w224 -> [w232] mode=indexing
              tunnel: [w231] -> w223 mode=indexing
              tunnel: [w230] -> w222 mode=indexing
              n127 = Index Array(array=w235, index=w232) -> (element=w234:timestamp)
              n128 = call "Signalverlaeufe in Graphen Umladen.vi"("Mittelwertdaten"=w236, "Gas-Auswahl"=w232, "t0"=w234, "Werte"=w233) -> ("Konzentration"=w230:sgl, "Waveform"=w231:waveform(dbl))  [unwired: 3 in, 3 out]
            }
            "Graph" <- w223
            n129 = Index Array(array=w222) -> (element #1=→"Komponente 1:":sgl, element #2=→"Komponente 2:":sgl, element #3=→"Komponente 3:":sgl, element #4=→"Komponente 4:":sgl, element #5=→"Interferent 1: 2":sgl, element #6=→"Interferent 2: 2":sgl, element #7=→"Interferent 3: 2":sgl, element #8=→"Interferent 4:":sgl)  [unwired: 8 in]
          }
          frame "Result" {
          }
        }
        n130 = call "Wertaenderung Gasliste.vi"("Aktion"=Aktion_Wertaenderung_Gasliste."lesen") -> ("Tests"=w195:T24)  [unwired: 13 in, 1 out]
        n131 = Unbundle By Name(w191) -> ("Interference 366 läuft"=w192:bool)
        n132 = Unbundle By Name(w195) -> ("Interference 366 läuft"=w194:bool)
        n133 = call "Test Status.vi"("Interference 366 läuft"=w197, "Aktion"=Aktion_Test_Status."Interference 366") -> ()  [unwired: 10 in, 4 out]
        n134 = case shown="True" w197 {
          tunnel: [_ w244] -> w207
          tunnel: [Aktion_Test."ini" ("Aktion") w243] -> w204
          tunnel: w203 -> [_ w242]
          tunnel: [_ w241] -> w202
          tunnel: [_ w240] -> w201
          tunnel: [_ w239] -> w200
          frame False {
          }
          frame True {
            n135 = call "VI Test.vi"("Aktion"=w242) -> ("Status Test"=w244:string, "Fertig"=w238:bool, "Aktion"=w243:T9, "Test"=w240:dbl, "Warten"=w239:dbl)  [unwired: 5 in, 1 out]
            n136 = Not(x=w238) -> (.not. x?=w241:bool)
            n137 = case shown="True" w238 {
              frame False {
              }
              frame True {
                n138 = property on="Registerkarte" class="RKElem (strikt)"("Val(Sgnl)"=T1."Result" ("Registerkarte")) -> (error out=w245:errorcluster)  [unwired: 2 in, 1 out]
                n139 = call "FGV Interference.vi"("error in (no error)"=w245, "Aktion FGV Interference"=Aktion_FGV_Interference."Lesen") -> ("Tabelle"=w248:T6[][])  [unwired: 8 in, 5 out]
                n140 = local write "LIN Ausgabetabelle"(w248) -> ()
              }
            }
          }
        }
        "Testdauer" <- w201
        "Stabilisierungszeit" <- w200
        n141 = case shown="True" w192 {
          selector: w192 -> [_ w209]
          frame False {
          }
          frame True {
            n142 = property on="Systemeinstellung" class="Bool. (strikt)"("Val(Sgnl)"=w209) -> (error out=w210:errorcluster)  [unwired: 2 in, 1 out]
            n143 = call <vilib>:"Clear Errors.vi"("error in (no error)"=w210) -> ()  [unwired: 5 in, 2 out]
          }
        }
        n144 = case shown="True" w194 {
          frame False {
          }
          frame True {
            n145 = property on="Gasliste vergleichen" class="Bool."("Val(Sgnl)"=TRUE) -> (error out=w212:errorcluster)  [unwired: 2 in, 1 out]
            n146 = call <vilib>:"Clear Errors.vi"("error in (no error)"=w212) -> ("error out"=w211:errorcluster)  [unwired: 5 in, 1 out]
            n147 = flat-sequence {
              tunnel: w211 -> [_]
              frame #0 {
              }
            }
          }
        }
        n148 = Empty String/Path?(string/path=w207) -> (empty?=w208:bool)
        n149 = case shown="False" w208 {
          tunnel: w205 -> [w249 w252]
          tunnel: w207 -> [w251 _]
          tunnel: [w250 w252] -> w206
          frame False {
            n150 = call "Strings und Zeitstempel verknuepfen.vi"("String 1 hinzufügen"=w251, "Eingagns String"=w249) -> ("Verknüpfter String"=w250:string)  [unwired: 9 in]
          }
          frame True {
          }
        }
      }
      event "Gasliste vergleichen": Value Change {
        n151 = event-data() -> ()  [unwired: 1 in, 1 out]
        n152 = stacked-sequence {
          frame #0 {
            n153 = call "FGV Gasliste.vi"("Aktionen"=FGV_FT-IR_Gasliste_Aktionen."lesen") -> ("Aktuelle Gasliste gesamt"=w261:T6[])  [unwired: 8 in, 2 out]
            n154 = for {
              tunnel: w261 -> [w294] mode=indexing
              tunnel: w261 -> [w293]
              tunnel: [w333] -> w269 mode=indexing if=w332
              tunnel: [w290] -> w273 mode=indexing if=w332
              tunnel: [w330] -> w270 mode=indexing if=w331
              tunnel: [w290] -> w274 mode=indexing if=w331
              tunnel: [w323] -> w271 mode=indexing if=w322
              tunnel: [w290] -> w275 mode=indexing if=w322
              tunnel: [w320] -> w278 mode=indexing if=w321
              tunnel: [w290] -> w282 mode=indexing if=w321
              tunnel: [w313] -> w279 mode=indexing if=w291
              tunnel: [w290] -> w283 mode=indexing if=w291
              tunnel: [w312] -> w280 mode=indexing if=w299
              tunnel: [w306] -> w272 mode=indexing if=w305
              tunnel: [w290] -> w276 mode=indexing if=w305
              tunnel: [w301] -> w277 mode=indexing if=w300
              tunnel: [w290] -> w281 mode=indexing if=w300
              tunnel: [w290] -> w284 mode=indexing if=w299
              tunnel: [w292] -> w286 mode=indexing if=w289
              tunnel: [w290] -> w288 mode=indexing if=w289
              i -> [w290]
              n155 = Search/Split String(string=w294, search string/char (-)="CH4" ("Such-String/-Zeichen (-)")) -> (match + rest of string=w335:T6)  [unwired: 1 in, 2 out]
              n156 = Search/Split String(string=w294, search string/char (-)="Ethane" ("Such-String/-Zeichen (-)")) -> (match + rest of string=w328:T6)  [unwired: 1 in, 2 out]
              n157 = Search/Split String(string=w294, search string/char (-)="NMHC" ("Such-String/-Zeichen (-)")) -> (match + rest of string=w325:T6)  [unwired: 1 in, 2 out]
              n158 = Search/Split String(string=w294, search string/char (-)="NMNEHC" ("Such-String/-Zeichen (-)")) -> (match + rest of string=w308:T6)  [unwired: 1 in, 2 out]
              n159 = Search/Split String(string=w294, search string/char (-)="CO2" ("Such-String/-Zeichen (-)")) -> (match + rest of string=w303:T6)  [unwired: 1 in, 2 out]
              n160 = Search/Split String(string=w294, search string/char (-)="H2O" ("Such-String/-Zeichen (-)")) -> (match + rest of string=w318:T6)  [unwired: 1 in, 2 out]
              n161 = Search/Split String(string=w294, search string/char (-)="CH4" ("Such-String/-Zeichen (-)")) -> (match + rest of string=w315:T6)  [unwired: 1 in, 2 out]
              n162 = Search/Split String(string=w294, search string/char (-)="Ethane" ("Such-String/-Zeichen (-)")) -> (match + rest of string=w310:T6)  [unwired: 1 in, 2 out]
              n163 = Search/Split String(string=w294, search string/char (-)="Propane" ("Such-String/-Zeichen (-)")) -> (match + rest of string=w296:T6)  [unwired: 1 in, 2 out]
              n164 = Empty String/Path?(string/path=w335) -> (empty?=w336:bool)
              n165 = Empty String/Path?(string/path=w328) -> (empty?=w327:bool)
              n166 = Empty String/Path?(string/path=w325) -> (empty?=w326:bool)
              n167 = Empty String/Path?(string/path=w308) -> (empty?=w307:bool)
              n168 = Empty String/Path?(string/path=w303) -> (empty?=w304:bool)
              n169 = Empty String/Path?(string/path=w318) -> (empty?=w317:bool)
              n170 = Empty String/Path?(string/path=w315) -> (empty?=w316:bool)
              n171 = Empty String/Path?(string/path=w310) -> (empty?=w309:bool)
              n172 = Empty String/Path?(string/path=w296) -> (empty?=w295:bool)
              n173 = Not(x=w336) -> (.not. x?=w332:bool)
              n174 = Not(x=w327) -> (.not. x?=w331:bool)
              n175 = Not(x=w326) -> (.not. x?=w322:bool)
              n176 = Not(x=w307) -> (.not. x?=w305:bool)
              n177 = Not(x=w304) -> (.not. x?=w300:bool)
              n178 = Not(x=w317) -> (.not. x?=w321:bool)
              n179 = Not(x=w316) -> (.not. x?=w291:bool)
              n180 = Not(x=w309) -> (.not. x?=w299:bool)
              n181 = Not(x=w295) -> (.not. x?=w289:bool)
              n182 = Index Array(array=w293, index=w290) -> (element=w333:T6)
              n183 = Index Array(array=w293, index=w290) -> (element=w330:T6)
              n184 = Index Array(array=w293, index=w290) -> (element=w323:T6)
              n185 = Index Array(array=w293, index=w290) -> (element=w306:T6)
              n186 = Index Array(array=w293, index=w290) -> (element=w301:T6)
              n187 = Index Array(array=w293, index=w290) -> (element=w320:T6)
              n188 = Index Array(array=w293, index=w290) -> (element=w313:T6)
              n189 = Index Array(array=w293, index=w290) -> (element=w312:T6)
              n190 = Index Array(array=w293, index=w290) -> (element=w292:T6)
            }
            n191 = Build Array (concatenate)(w280, w286) -> (w285:T6[])
            n192 = Build Array (concatenate)(w284, w288) -> (w287:i32[])
            n193 = property on="CH4:" class="Ring (strikt)"("Strings []"=w269) -> (error out=w259:errorcluster)  [unwired: 2 in, 1 out]
            n194 = property on="Ethane:" class="Ring (strikt)"("Strings []"=w270) -> (error out=w268:errorcluster)  [unwired: 2 in, 1 out]
            n195 = property on="NMHC:" class="Ring (strikt)"("Strings []"=w271) -> (error out=w265:errorcluster)  [unwired: 2 in, 1 out]
            n196 = property on="NMNEHC:" class="Ring (strikt)"("Strings []"=w272) -> (error out=w264:errorcluster)  [unwired: 2 in, 1 out]
            n197 = property on="Interferent 1: CO2" class="Ring (strikt)"("Strings []"=w277) -> (error out=w263:errorcluster)  [unwired: 2 in, 1 out]
            n198 = property on="Interferent 2: H2O" class="Ring (strikt)"("Strings []"=w278) -> (error out=w262:errorcluster)  [unwired: 2 in, 1 out]
            n199 = property on="Interferent 3: CH4" class="Ring (strikt)"("Strings []"=w279) -> (error out=w267:errorcluster)  [unwired: 2 in, 1 out]
            n200 = property on="Interferent 4: C2H6 / C3H8" class="Ring (strikt)"("Strings []"=w285) -> (error out=w258:errorcluster)  [unwired: 2 in, 1 out]
            n201 = Build Array(w273, w274, w275, w276, w281, w282, w283, w287) -> (w260:i32[][])
            n202 = call "Index uebersetzen.vi"("Aktion"=Aktion_Index_uebersetzten."schreiben", "Array"=w260) -> ()  [unwired: 8 in, 2 out]
            n203 = Merge Errors(w259, w268, w265, w264, w263, w262, w267, w258) -> (w256:errorcluster)
            n204 = call <vilib>:"Clear Errors.vi"("error in (no error)"=w256) -> ()  [unwired: 5 in, 2 out]
          }
          frame #1 {
            n205 = flat-sequence {
              tunnel: [w401] -> w373
              tunnel: w373 -> [w421]
              frame #0 {
                n206 = call "Index uebersetzen.vi"("Aktion"=Aktion_Index_uebersetzten."auswerten") -> ("Komponenten"=w396:T16)  [unwired: 9 in, 1 out]
                n207 = Unbundle By Name(w396) -> ("Komponente"=w392:T6, "Komponente 2"=w390:T6, "Komponente 3"=w391:T6, "Komponente 4"=w389:T6, "Interferent 1"=w397:T6, "Interferent 2"=w398:T6, "Interferent 3"=w394:T6, "Interferent 4"=w393:T6)
                n208 = local write "Komponente 1S:"(w392) -> ()
                n209 = local write "Komponente 2S:"(w390) -> ()
                n210 = local write "Komponente 3S:"(w391) -> ()
                n211 = local write "Komponente 4S:"(w389) -> ()
                n212 = local write "Interferent 1:"(w397) -> ()
                n213 = local write "Interferent 2:"(w398) -> ()
                n214 = local write "Interferent 3:"(w394) -> ()
                n215 = local write "Interferent 4:"(w393) -> ()
              }
              frame #1 {
                n216 = control-ref of="Komponente:"() -> (w411:refnum<vi>)
                n217 = control-ref of="Komponente 1:"() -> (w416:refnum<vi>)
                n218 = control-ref of="Komponente 2:"() -> (w417:refnum<vi>)
                n219 = control-ref of="Komponente 3:"() -> (w418:refnum<vi>)
                n220 = control-ref of="Komponente 4:"() -> (w399:refnum<vi>)
                n221 = control-ref of="Interferent 1: 2"() -> (w408:refnum<vi>)
                n222 = control-ref of="Interferent 2: 2"() -> (w407:refnum<vi>)
                n223 = control-ref of="Interferent 3: 2"() -> (w406:refnum<vi>)
                n224 = control-ref of="Interferent 3: 3"() -> (w413:refnum<vi>)
                n225 = control-ref of="CH4:"() -> (w414:refnum<vi>)
                n226 = control-ref of="Ethane:"() -> (w415:refnum<vi>)
                n227 = control-ref of="NMHC:"() -> (w402:refnum<vi>)
                n228 = control-ref of="NMNEHC:"() -> (w403:refnum<vi>)
                n229 = control-ref of="Interferent 1: CO2"() -> (w404:refnum<vi>)
                n230 = control-ref of="Interferent 2: H2O"() -> (w405:refnum<vi>)
                n231 = control-ref of="Interferent 3: CH4"() -> (w412:refnum<vi>)
                n232 = control-ref of="Interferent 4: C2H6 / C3H8"() -> (w400:refnum<vi>)
                n233 = Build Array(w411) -> (w410:refnum<vi>[])
                n234 = Build Array(w414, w415, w402, w403, w404, w405, w412, w400) -> (w401:refnum<vi>[])
                n235 = Build Array(w416, w417, w418, w399, w408, w407, w406, w413) -> (w409:refnum<vi>[])
                n236 = call "dynEinheiten.vi"("Komponenten Ref."=w401, "Sollwert Ref."=w409) -> ()  [unwired: 10 in]
                n237 = call "dynEinheiten.vi"("Komponenten Ref."=w401, "Sollwert Ref."=w401) -> ()  [unwired: 10 in]
                n238 = call "dynEinheiten.vi"("Komponenten Ref."=w401, "Sollwert Ref."=w410) -> ()  [unwired: 10 in]
              }
              frame #2 {
                n239 = for {
                  tunnel: w421 -> [w423] mode=indexing
                  tunnel: [w422] -> w419 mode=indexing
                  n240 = property class="Ring (strikt)"(reference=w423) -> ("Caption.Text"=w422:string)  [unwired: 1 in, 2 out]
                }
                n241 = call "FGV Interference.vi"("Êinheiten"=w419, "Aktion FGV Interference"=Aktion_FGV_Interference."Einheiten") -> ()  [unwired: 8 in, 6 out]
              }
            }
            n242 = Unbundle By Name("TestKonfig") -> ("Komp 1 aktiv:"=w369:bool, "Komp 2 aktiv:"=w368:bool, "Komp 3 aktiv:"=w367:bool, "Komp 4 aktiv:"=w341:bool, "Inter 1 aktiv"=w366:bool, "Inter 2 aktiv"=w343:bool, "Inter 3 aktiv"=w365:bool, "Inter 4 aktiv"=w364:bool)
            n243 = control-ref of="Komponente 1:"() -> (w358:refnum<vi>)
            n244 = control-ref of="Komponente 2:"() -> (w357:refnum<vi>)
            n245 = control-ref of="Komponente 3:"() -> (w356:refnum<vi>)
            n246 = control-ref of="Komponente 4:"() -> (w340:refnum<vi>)
            n247 = control-ref of="Interferent 1: 2"() -> (w360:refnum<vi>)
            n248 = control-ref of="Interferent 2: 2"() -> (w361:refnum<vi>)
            n249 = control-ref of="Interferent 3: 2"() -> (w362:refnum<vi>)
            n250 = control-ref of="Interferent 3: 3"() -> (w359:refnum<vi>)
            n251 = control-ref of="Komponente 1S:"() -> (w355:refnum<vi>)
            n252 = control-ref of="Komponente 2S:"() -> (w354:refnum<vi>)
            n253 = control-ref of="Komponente 3S:"() -> (w339:refnum<vi>)
            n254 = control-ref of="Komponente 4S:"() -> (w338:refnum<vi>)
            n255 = control-ref of="Interferent 1:"() -> (w353:refnum<vi>)
            n256 = control-ref of="Interferent 2:"() -> (w352:refnum<vi>)
            n257 = control-ref of="Interferent 3:"() -> (w351:refnum<vi>)
            n258 = control-ref of="Interferent 4:"() -> (w350:refnum<vi>)
            n259 = call "FGV Interference.vi"("TestKonfig"="TestKonfig", "Aktion FGV Interference"=Aktion_FGV_Interference."TestKonfig") -> ()  [unwired: 8 in, 6 out]
            n260 = property on="Graph" class="SVDiagr (strikt)"("LegNumRows"=u32 8 ("Legende:Zeilenanzahl")) -> (error out=w371:errorcluster)  [unwired: 2 in, 1 out]
            n261 = Build Array(w358, w357, w356, w340, w360, w361, w362, w359) -> (w349:refnum<vi>[])
            n262 = Build Array(w355, w354, w339, w338, w353, w352, w351, w350) -> (w348:refnum<vi>[])
            n263 = Build Array(w369, w368, w367, w341, w366, w343, w365, w364) -> (w344:bool[])
            n264 = for {
              tunnel: w344 -> [w374] mode=indexing
              tunnel: w349 -> [w381] mode=indexing
              tunnel: w348 -> [w380] mode=indexing
              tunnel: [w379] -> w347 mode=indexing
              tunnel: [w378] -> w346 mode=indexing
              n265 = Select(t=T13."Enabled" ("Deaktiviert"), s=w374, f=T13."Disabled and Grayed Out" ("Deaktiviert")) -> (s? t:f=w375:T13)
              n266 = property class="DigWert (strikt)"(reference=w381, "DisabledEnum"=w375) -> (error out=w379:errorcluster)  [unwired: 1 in, 1 out]
              n267 = property class="Str (strikt)"(reference=w380, "DisabledEnum"=w375) -> (error out=w378:errorcluster)  [unwired: 1 in, 1 out]
            }
            n268 = for {
              shift-right: [w385] -> w363
              shift-left: w371 -> [w384]
              tunnel: w344 -> [w382] mode=indexing
              i -> [w383]
              n269 = property on="Graph" class="SVDiagr (strikt)"(error in=w384, "Active Plot"=w383) -> (error out=w386:errorcluster)  [unwired: 1 in, 1 out]
              n270 = property on="Graph" class="SVDiagr (strikt)"(error in=w386, "Plot.Visible?"=w382) -> (error out=w387:errorcluster)  [unwired: 1 in, 1 out]
              n271 = property on="Graph" class="SVDiagr (strikt)"(error in=w387, "Active Plot"=w383) -> (error out=w388:errorcluster)  [unwired: 1 in, 1 out]
              n272 = property on="Graph" class="SVDiagr (strikt)"(error in=w388, "Plot.Visible?"=w382) -> (error out=w385:errorcluster)  [unwired: 1 in, 1 out]
            }
            n273 = Merge Errors(w347, w346) -> (w345:errorcluster)
            n274 = call <vilib>:"Clear Errors.vi"("error in (no error)"=w363) -> ()  [unwired: 5 in, 2 out]
            n275 = call <vilib>:"Clear Errors.vi"("error in (no error)"=w345) -> ()  [unwired: 5 in, 2 out]
            n276 = call "Wertaenderung Gasliste.vi"("Aktion"=Aktion_Wertaenderung_Gasliste."Interference 366 inaktiv") -> ()  [unwired: 13 in, 2 out]
          }
        }
      }
      event "Systemeinstellung": Value Change {
        n277 = event-data() -> ()  [unwired: 1 in, 6 out]
        n278 = stacked-sequence {
          frame #0 {
          }
          frame #1 {
            n279 = control-ref of="Analysator"() -> (w427:refnum<vi>)
            n280 = call "Analysator initialisieren.vi"("Referenz Analysator"=w427) -> ()  [unwired: 9 in, 2 out]
          }
          frame #2 {
            n281 = call "Wertaenderung Systemeinstellungen.vi"("Aktion"=Aktion_Wertaenderung_Gasliste."Interference 366 inaktiv") -> ()  [unwired: 13 in, 2 out]
            n282 = local write "Systemeinstellung"(FALSE ("Systemeinstellung")) -> ()
          }
        }
      }
      event Value Change {
        n283 = event-data() -> ()  [unwired: 1 in, 1 out]
        n284 = call "FGV Interference.vi"("TestSetting"="TestSetting", "Aktion FGV Interference"=Aktion_FGV_Interference."TestSetting") -> ("error out"=w430:errorcluster)  [unwired: 8 in, 5 out]
        n285 = call "FGV Interference.vi"("error in (no error)"=w430, "Aktion FGV Interference"=Aktion_FGV_Interference."Speichern") -> ()  [unwired: 8 in, 6 out]
      }
      event "Test Start": Value Change {
        n286 = event-data() -> ()  [unwired: 1 in, 6 out]
        n287 = call "Test Status.vi"("Aktion"=Aktion_Test_Status."lesen") -> ("Tests sperren"=w437:bool)  [unwired: 11 in, 3 out]
        n288 = case shown="False" w437 {
          tunnel: [TRUE FALSE] -> w441
          tunnel: w438 -> [_ w443]
          frame False {
          }
          frame True {
            n289 = call "Texte in VIs uebersetzen.vi"("Sprachliste"=w443, "String zum Übersetzen"="Anderer Test läuft gerade.\nBitte etwas Geduld." ("Nachricht")) -> ("String zum Übersetzen"=w444:string)  [unwired: 9 in, 4 out]
            n290 = One Button Dialog(message=w444, button name ("OK")="OK" ("Schaltflächentext (\"OK\")")) -> ()  [unwired: 1 out]
          }
        }
      }
      event "Abbrechen": Value Change {
        n291 = event-data() -> ()  [unwired: 1 in, 3 out]
        n292 = call "Test Status.vi"("Aktion"=Aktion_Test_Status."lesen") -> ("Aktive Tests"=w451:T24, "Tests sperren"=w449:bool)  [unwired: 11 in, 2 out]
        n293 = Unbundle By Name(w451) -> ("Interference 366 läuft"=w450:bool)
        n294 = And(x=w450, y=w449) -> (x .and. y?=w448:bool)
        n295 = case shown="True" w448 {
          tunnel: [w458 w466] -> w457
          tunnel: w456 -> [w458 w465]
          tunnel: w453 -> [_ w459]
          frame False {
          }
          frame True {
            n296 = call "FGV-Funktionstasten.vi"("Herkunft"="Interference Test", "Zustand"=Zustaende."Standby", "Aktion"=Funktionstasten-Aktion."Zustand setzen") -> ()  [unwired: 5 in, 8 out]
            n297 = call "Texte in VIs uebersetzen.vi"("Sprachliste"=w459, "String zum Übersetzen"="Test abgebrochen" ("String 1 hinzufügen")) -> ("String zum Übersetzen"=w460:string)  [unwired: 9 in, 4 out]
            n298 = call "Strings und Zeitstempel verknuepfen.vi"("String 1 hinzufügen"=w460, "Eingagns String"=w465) -> ("Verknüpfter String"=w466:string)  [unwired: 9 in]
          }
        }
      }
      event "Daten löschen": Value Change {
        n299 = event-data() -> ()  [unwired: 1 in, 3 out]
        n300 = flat-sequence {
          frame #0 {
            n301 = call "FGV Interference.vi"("Aktion FGV Interference"=Aktion_FGV_Interference."löschen") -> ("Tabelle"=w470:T6[][])  [unwired: 9 in, 5 out]
            n302 = local write "LIN Ausgabetabelle"(w470) -> ()
          }
          frame #1 {
            n303 = call "Auswerten.vi"() -> ("Konzentration Komponente"=w471:dbl, "Komponente:"=w472:T6, "max. Flow Weighted Mean:"=w473:T6, "Konzentration FlowWeightedMean"=w474:dbl, "[%]"=w475:dbl)  [unwired: 6 in, 1 out]
            n304 = local write "[%]"(w475) -> ()
            n305 = local write "Konzentration FlowWeightedMean"(w474) -> ()
            n306 = local write "max. Flow Weighted Mean:"(w473) -> ()
            n307 = local write "Komponente:"(w472) -> ()
            n308 = local write "Konzentration Komponente"(w471) -> ()
          }
          frame #2 {
            n309 = control-ref of="LIN Ausgabetabelle"() -> (w477:refnum<vi>)
            n310 = call "Zeile faerben.vi"("Anzahl"=5, "Table (Eingang)"=w477) -> ()  [unwired: 9 in, 1 out]
          }
        }
      }
      event "Print to PDF": Value Change {
        n311 = event-data() -> ()  [unwired: 1 in, 1 out]
        n312 = call "FGV Interference.vi"("Aktion FGV Interference"=Aktion_FGV_Interference."Lesen") -> ("TestSetting"=w488:T2)  [unwired: 9 in, 5 out]
        n313 = Unbundle By Name(w488) -> ("Pfad:"=w487:path, "Textname:"=w486:string)
        n314 = Concatenate Strings(w486, ".pdf") -> (w494:string)
        n315 = Build Path(base path=w487, name or relative path=w494) -> (appended path=w478:path)
        n316 = disable-structure shown="BullZip==FALSE, Standard" {
          disable-tunnel: w478 -> [w503 _]
          disable-tunnel: [w502 _] -> w480
          frame condition #0 {
            n317 = call "Save to PDF File using BullZip 2009.vi"("Save PDF File Path"=w503) -> ("error out"=w502:errorcluster)  [unwired: 10 in]
          }
          frame condition #1 (active) {
          }
        }
        n318 = disable-structure shown="Aktiviert" {
          disable-tunnel: w480 -> [w496 w499]
          disable-tunnel: [w495 w498] -> w479
          disable-tunnel: w478 -> [_ w497]
          frame Disabled {
            n319 = call "PDF Protokoll EPA1065_InterferenceVerification.vi"("error in (no error)"=w496) -> ("error out"=w495:errorcluster)  [unwired: 10 in]
          }
          frame Enabled {
            # "#PDF_Interface"
            n320 = call "PDF_Interface_PDF Protokoll EPA1065_InterferenceVerification.vi"("error in (no error)"=w499, "Save PDF File Path"=w497) -> ("error out"=w498:errorcluster)  [unwired: 9 in]
          }
        }
        n321 = case shown="Fehler" w479 {
          tunnel: ["Daten gespeichert!" ("String") "Fehler beim schreiben der Daten" ("String")] -> w484
          frame No Error {
          }
          frame Error {
          }
        }
        n322 = call <vilib>:"Clear Errors.vi"("error in (no error)"=w479) -> ()  [unwired: 5 in, 2 out]
        n323 = call "Tabelle in die einzelnen Seiten zerlegen.vi"("Aktion"=FGV_Aktion_Tabelle_zerlegen."vereinzeln", "Index (Seite)"=38) -> ("Sprachliste"=w483:string[][])  [unwired: 7 in, 2 out]
        n324 = call "Texte in VIs uebersetzen.vi"("Sprachliste"=w483, "String zum Übersetzen"=w484) -> ("String zum Übersetzen"=w485:string)  [unwired: 9 in, 4 out]
        n325 = One Button Dialog(message=w485) -> ()  [unwired: 1 in, 1 out]
      }
      event "Save to file": Value Change {
        n326 = event-data() -> ()  [unwired: 1 in, 1 out]
        n327 = call "FGV Interference.vi"("Aktion FGV Interference"=Aktion_FGV_Interference."Lesen") -> ("TestSetting"=w522:T2)  [unwired: 9 in, 5 out]
        n328 = Unbundle By Name(w522) -> ("Pfad:"=w521:path, "Textname:"=w520:string)
        n329 = Concatenate Strings(w520, ".txt") -> (w525:string)
        n330 = Build Path(base path=w521, name or relative path=w525) -> (appended path=w509:path)
        n331 = Open/Create/Replace File(file path (use dialog)=w509, operation (0:open)=T22."replace or create with confirmation" ("Operation (0:Öffnen)")) -> (refnum out=w511:refnum<file>, error out=w512:errorcluster)  [unwired: 4 in, 1 out]
        n332 = call "Interference 1065-366 Textfile.vi"() -> ("Tabelle für Textdatei"=w507:string[])  [unwired: 11 in]
        n333 = Write to Text File(file (use dialog)=w511, text=w507, error in=w512) -> (refnum out=w514:refnum<file>, error out=w508:errorcluster)  [unwired: 1 in, 1 out]
        n334 = Close File(refnum=w514, error in=w508) -> (error out=w513:errorcluster)  [unwired: 1 out]
        n335 = call <vilib>:"Clear Errors.vi"("error in (no error)"=w513) -> ()  [unwired: 5 in, 2 out]
        n336 = case shown="Fehler" w508 {
          tunnel: ["Daten gespeichert!" ("String") "Fehler beim schreiben der Daten" ("String")] -> w518
          frame No Error {
          }
          frame Error {
          }
        }
        n337 = call "Tabelle in die einzelnen Seiten zerlegen.vi"("Aktion"=FGV_Aktion_Tabelle_zerlegen."vereinzeln", "Index (Seite)"=38) -> ("Sprachliste"=w517:string[][])  [unwired: 7 in, 2 out]
        n338 = call "Texte in VIs uebersetzen.vi"("Sprachliste"=w517, "String zum Übersetzen"=w518) -> ("String zum Übersetzen"=w519:string)  [unwired: 9 in, 4 out]
        n339 = One Button Dialog(message=w519) -> ()  [unwired: 1 in, 1 out]
      }
      event "Speichern": Value Change {
        n340 = event-data() -> ()  [unwired: 1 in, 6 out]
        n341 = call "FGV Interference.vi"("Aktion FGV Interference"=Aktion_FGV_Interference."Speichern") -> ()  [unwired: 9 in, 6 out]
      }
      event "Graph löschen": Value Change {
        n342 = event-data() -> ()  [unwired: 1 in, 3 out]
        n343 = property on="Graph" class="SVDiagr (strikt)"("History Data"=waveform(dbl)[][] [] ("Historiendaten")) -> (error out=w536:errorcluster)  [unwired: 2 in, 1 out]
        n344 = call <vilib>:"Clear Errors.vi"("error in (no error)"=w536) -> ()  [unwired: 5 in, 2 out]
        n345 = call "FGV Messdaten.vi"("Aktionen"=Aktionen_FGV_Messdaten."löschen") -> ()  [unwired: 6 in, 9 out]
      }
      event "Registerkarte": Value Change {
        n346 = event-data() -> ()  [unwired: 1 in, 6 out]
        n347 = flat-sequence {
          tunnel: [w572] -> w555
          tunnel: [w566] -> w542
          frame #0 {
            n348 = control-ref of="LIN Ausgabetabelle"() -> (w557:refnum<vi>)
            n349 = call "Zeile faerben.vi"("Anzahl"=5, "Table (Eingang)"=w557) -> ()  [unwired: 9 in, 1 out]
          }
          frame #1 {
            n350 = call "FGV Interference.vi"("Aktion FGV Interference"=Aktion_FGV_Interference."Lesen") -> ("Tabelle"=w572:T6[][])  [unwired: 9 in, 5 out]
            n351 = control-ref of="LIN Ausgabetabelle"() -> (w577:refnum<vi>)
            n352 = control-ref of="max. Flow Weighted Mean:"() -> (w579:refnum<vi>)
            n353 = control-ref of="Komponente:"() -> (w578:refnum<vi>)
            n354 = call "Auswerten.vi"("LIN Ausgabetabelle"=w577, "Komponente:"=w578, "max. Flow Weighted Mean:"=w579) -> ("Konzentration Komponente"=→"Konzentration Komponente":dbl, "Komponente:"=→"Komponente:":T6, "max. Flow Weighted Mean:"=→"max. Flow Weighted Mean:":T6, "Konzentration FlowWeightedMean"=→"Konzentration FlowWeightedMean":dbl, "Limit in ppm"=w563:dbl, "[%]"=w564:dbl)  [unwired: 3 in]
            "[%]" <- w564
            "Grenze in ppm:" <- w563
            n355 = Greater Or Equal?(x=w563, y=1.0) -> (x >= y?=w561:bool)
            n356 = Greater Or Equal?(x=w564, y=-2.0) -> (x >= y?=w560:bool)
            n357 = And(x=w561, y=w560) -> (x .and. y?=w559:bool)
            n358 = disable-structure shown="Aktiviert" {
              disable-tunnel: [w582 w583] -> w570
              disable-tunnel: w564 -> [w581 w583]
              frame Disabled {
                n359 = Absolute Value(x=w581) -> (abs(x)=w582:dbl)
              }
              frame Enabled {
              }
            }
            n360 = property on="[%]" class="DigWert (strikt)"("Visible"=w559) -> (error out=w558:errorcluster)  [unwired: 2 in, 1 out]
            n361 = Less Or Equal?(x=w570, y=2.0) -> (x <= y?=w568:bool)
            n362 = Not A Number/Path/Refnum?(number/path/refnum=w570) -> (NaN/Path/Refnum?=w569:bool)
            n363 = call <vilib>:"Clear Errors.vi"("error in (no error)"=w558) -> ()  [unwired: 5 in, 2 out]
            n364 = Not(x=w569) -> (.not. x?=w567:bool)
            n365 = And(x=w567, y=w568) -> (x .and. y?=w566:bool)
          }
        }
        n366 = property on="Tabelle 3" class="Tbl (strikt)"("Active Cell"=T23 {"Row"=0, "Column"=1} ("Aktive Zelle:Aktive Zelle")) -> (error out=w548:errorcluster)  [unwired: 2 in, 1 out]
        n367 = Select(t=u32 6618880, s=w542, f=u32 16711680) -> (s? t:f=w549:u32)
        n368 = property on="Tabelle 3" class="Tbl (strikt)"(error in=w548, "Cell BG Color"=w549) -> (error out=w543:errorcluster)  [unwired: 1 in, 1 out]
        n369 = property on="Tabelle 3" class="Tbl (strikt)"(error in=w543, "Active Cell"=T23 {"Row"=0, "Column"=1} ("Aktive Zelle:Aktive Zelle")) -> ()  [unwired: 1 in, 2 out]
        n370 = Select(t=string[][] [["EPA §1065.366 Interference verification"], ["Passed"]] ("Tabelle 3"), s=w542, f=string[][] [["EPA §1065.366 Interference verification"], ["NOT Passed"]] ("Tabelle 3")) -> (s? t:f=w539:string[][])
        n371 = call "Texte in VIs uebersetzen.vi"("Sprachliste"=w540, "2D String-Array zum Übersetzen"=w539) -> ("2D String-Array zum Übersetzen"=w541:string[][])  [unwired: 9 in, 4 out]
        n372 = Transpose 2D Array(2D array=w541) -> (transposed array=→"Tabelle 3":string[][])
        "LIN Ausgabetabelle" <- w555
      }
    }
    "Status" <- w183
    n373 = Not Equal?(x=w185, y=w183) -> (x != y?=w184:bool)
    n374 = case shown="False" w184 {
      frame False {
      }
      frame True {
        n375 = property on="Status" class="Str"("Text.Scroll Position"=u32 9999 ("Text.Anzeigeposition")) -> (error out=w585:errorcluster)  [unwired: 2 in, 1 out]
        n376 = call <vilib>:"Clear Errors.vi"("error in (no error)"=w585) -> ()  [unwired: 5 in, 2 out]
      }
    }
  }
